vi "Main.vi"() -> ()   [LabVIEW 2017]
uses:
  type defs/action buttons.ctl
  type defs/mode buttons.ctl
  <vilib>/vision/Pattern Matching.llb/IMAQ GM Match Report.ctl
  type defs/states.ctl
  type defs/data.ctl
  <vilib>/vision/Image Controls.llb/IMAQ Image.ctl
  <vilib>/myRIO/Instrument Drivers/Onboard IO/PWM/typedefs/PWM Reference.ctl
  <vilib>/myRIO/Common/Instrument Driver Framework/Utilities/typedefs/myRIO Generic Hardware Reference.ctl
  <vilib>/myRIO/Common/Instrument Driver Framework/Utilities/typedefs/Hardware Version Enum.ctl
  <vilib>/myRIO/Common/Instrument Driver Framework/Utilities/typedefs/myRIO v1.0 Reference.ctl
  <vilib>/myRIO/Common/Instrument Driver Framework/Utilities/typedefs/Generic FPGA Reference.ctl
  <vilib>/myRIO/Common/Instrument Driver Framework/myRIO v1.0/PWM/typedefs/PWM Channels Enum.ctl
  <vilib>/myRIO/Instrument Drivers/Onboard IO/PWM/typedefs/PWM Configuration.ctl
  <vilib>/userdefined/High Color/nirio_resource_hc.ctl
  <vilib>/myRIO/Instrument Drivers/Onboard IO/DIO/typedefs/DIO Reference.ctl
  <vilib>/myRIO/Common/Instrument Driver Framework/myRIO v1.0/DIO/typedefs/DIO Channels List.ctl
  <vilib>/myRIO/Common/Instrument Driver Framework/myRIO v1.0/DIO/typedefs/DIO Channels Enum.ctl
  type defs/task.ctl
  <vilib>/myRIO/Common/Instrument Driver Framework/Utilities/vis/Is FPGA Ref Available.vi
  <vilib>/myRIO/Common/Instrument Driver Framework/myRIO v1.0/PWM/vis/myRIO v1.1 Open PWM.vi
  <vilib>/myRIO/Instrument Drivers/Onboard IO/PWM/vis/Set Duty Cycle and Frequency.vi
  <vilib>/myRIO/Common/Instrument Driver Framework/myRIO v1.0/DIO/vis/myRIO v1.1 Open DIO.vi
  <vilib>/myRIO/Instrument Drivers/Onboard IO/DIO/vis/Write.vi
  <vilib>/myRIO/Instrument Drivers/Onboard IO/DIO/vis/Read.vi
  <vilib>/myRIO/Common/Instrument Driver Framework/Utilities/vis/Validate Channels.vi
  <vilib>/myRIO/Common/Instrument Driver Framework/myRIO v1.0/PWM/vis/myRIO v1.0 Reserve PWM.vi
  <vilib>/myRIO/Common/Instrument Driver Framework/myRIO v1.0/DIO/vis/myRIO v1.0 Reserve DIO.vi
  <vilib>/myRIO/Common/Instrument Driver Framework/myRIO v1.0/UART/vis/myRIO v1.0 Close UART.vi
  <vilib>/myRIO/Common/Instrument Driver Framework/myRIO v1.0/PWM/vis/myRIO v1.0 Build MUX Configuration PWM.vi
  <vilib>/myRIO/Common/Instrument Driver Framework/myRIO v1.0/Resource Manager/vis/myRIO v1.0 Reserve Channel List.vi
  <vilib>/myRIO/Common/Instrument Driver Framework/myRIO v1.0/DIO/vis/myRIO v1.0 Build MUX Configuration DIO.vi
  <vilib>/myRIO/Common/Instrument Driver Framework/myRIO v1.0/Resource Manager/vis/myRIO v1.0 Create Configuration List.vi
  <vilib>/myRIO/Common/Instrument Driver Framework/myRIO v1.0/Resource Manager/vis/myRIO v1.0 Reserve Channel.vi
  <vilib>/myRIO/Common/Instrument Driver Framework/myRIO v1.0/Resource Manager/vis/myRIO v1.0 Unreserve Channel.vi
  <vilib>/myRIO/Common/Instrument Driver Framework/myRIO v1.0/Resource Manager/vis/myRIO v1.0 Build Mutex Name.vi
  <vilib>/Utility/VariantDataType/GetNumericInfo.vi
  <vilib>/Utility/error.llb/Error Cluster From Error Code.vi
  <vilib>/myRIO/Common/Instrument Driver Framework/myRIO v1.0/myRIO v1.1 Open.vi
  <vilib>/myRIO/Common/Instrument Driver Framework/Utilities/vis/IO Manager.vi
  <vilib>/myRIO/Common/Instrument Driver Framework/Utilities/vis/Configuration Manager.vi
  <vilib>/myRIO/Common/Instrument Driver Framework/myRIO v1.0/Resource Manager/vis/myRIO v1.0 Configure IO.vi
  <vilib>/myRIO/Common/Instrument Driver Framework/myRIO v1.0/myRIO v1.0 Close.vi
  <vilib>/myRIO/Common/Instrument Driver Framework/myRIO v1.0/PWM/vis/myRIO v1.0 Write PWM.vi
  <vilib>/myRIO/Common/Instrument Driver Framework/myRIO v1.0/DIO/vis/myRIO v1.0 Write DIO.vi
  <vilib>/myRIO/Common/Instrument Driver Framework/myRIO v1.0/DIO/vis/myRIO v1.0 Read DIO.vi
  <vilib>/myRIO/Common/Instrument Driver Framework/Utilities/vis/FPGA Ref Manager.vi
  <vilib>/myRIO/Common/Instrument Driver Framework/myRIO v1.0/myRIO v1.0 Reset FPGA.vi
  <vilib>/myRIO/Common/Instrument Driver Framework/myRIO v1.0/IRQ/vis/myRIO v1.0 IRQ Info FGV.vi
  <vilib>/myRIO/Common/Instrument Driver Framework/myRIO v1.0/IRQ/vis/myRIO v1.0 Timer IRQ Info FGV.vi
  <vilib>/myRIO/Common/Instrument Driver Framework/myRIO v1.0/IRQ/vis/myRIO v1.0 ISR Agent.vi
  <vilib>/myRIO/Express VI/Onboard IO/PWM/PWM Express VI.xnode
  <vilib>/myRIO/Instrument Drivers/Onboard IO/PWM/vis/myRIO PWM Open.xnode
  <vilib>/myRIO/Express VI/Onboard IO/DO/DO Express VI.xnode
  <vilib>/myRIO/Instrument Drivers/Onboard IO/DIO/vis/myRIO DIO Open.xnode
  <vilib>/myRIO/Express VI/Onboard Devices/LED/LED Express VI.xnode
  <vilib>/myRIO/Express VI/Onboard Devices/Button/Button Express VI.xnode
  <vilib>/vision/NI_Vision_Development_Module.lvlib
  <vilib>/myRIO/Instrument Drivers/Onboard IO/DIO/DIO.lvlib
  <vilib>/myRIO/Instrument Drivers/Onboard IO/PWM/PWM.lvlib
  <vilib>/myRIO/Instrument Drivers/Utilities/Utilities.lvlib
panel:
  in  "ROI Descriptor COLOR":T1={"Global Rectangle"=[86, 71, 180, 164], "Contours"=[{"ID"=enum."External", "Type"=3, "Coordinates"=[86, 71, 180, 164]}]} {"Contours"."Type" items=["No Selection", "Point", "Line", "Rectangle", "Oval", "Polygon", "Freehand Region", "Annulus", "Unused2", "Unused3", "Broken Line", "Freehand Line", "Rotated Rectangle"]}
  out "y0 (circle)":i32
  out "x0 (circle)":i32
  out "x1 (circle)":i32
  out "y1 (circle)":i32
  in  "divider (circle)":dbl=1.0
  out "error out 2":errorcluster
  out "___Test___":i32[](array[numeric])
  in  "Ball index":i32=1
  out "CircleRadius":dbl
  in  "Look at ball":bool
  in  "x = y?":bool
  in  "y":sgl=1.0
  out "Scale":sgl
  out "error out":errorcluster
  in  "Tab Control":enum32{"Motors", "Shape/Color", "Pattern"}(tab)
  in  "Left+":bool
  in  "Left-":bool
  in  "Right+":bool
  in  "Right-":bool
  in  "M+":bool
  in  "M-":bool
  in  "G+":bool
  in  "G-":bool
  in  "M_PWM":dbl=0.5
  in  "L_PWM":dbl=0.5
  in  "R_PWM":dbl=0.5
  in  "M+ (onGrab)":bool
  out "Circles Calibrated (Shape Detection 1)":T2(array[cluster]) {"Position"."Y" format="%.2f"; "Position"."X" format="%.2f"}
  out "Number of Matches (Shape Detection 1)":i32
  out "Color":i32
  in  "Circle Descriptor (Shape Detection 1)":cluster{"Min Radius":dbl, "Max Radius":dbl}={"Min Radius"=16.0, "Max Radius"=500.0}
  in  "Align X - t, Y - f":bool
  in  "grab time (ms)":u32
  out "Class (Particle Classification 1)":string
  out "y0":i32
  out "x0":i32
  out "x1":i32
  out "y1":i32
  out "Number of Matches (Geometric Matching 1)":i32
  out "Calibrated Matches (Geometric Matching 1)":T3[](array[typedef]) {"Correlation Score" format="%.2f"; "Target Template Curve Score" format="%.2f"; "Template Target Curve Score" format="%.2f"; "Bounding Box"."y" format="%.2f"; "Bounding Box"."x" format="%.2f"; "Position"."y" format="%.2f"; "Position"."x" format="%.2f"; "Score" format="%.2f"; "Scale" format="%.2f"; "Angle" format="%.2f"; "Occlusion %" format="%.2f"}
  out "curY":dbl
  out "curX":dbl
  out "Y is in range":bool
  out "X is in range":bool
  in  "defY":dbl=170.0
  in  "Range":dbl=40.0
  in  "defX":dbl=150.0
  in  "mode buttons":T4
  out "image display":T5(plugin-control)
  in  "action buttons":T6
  in  "Stop":bool
  # "Machine\nVision\nApp"
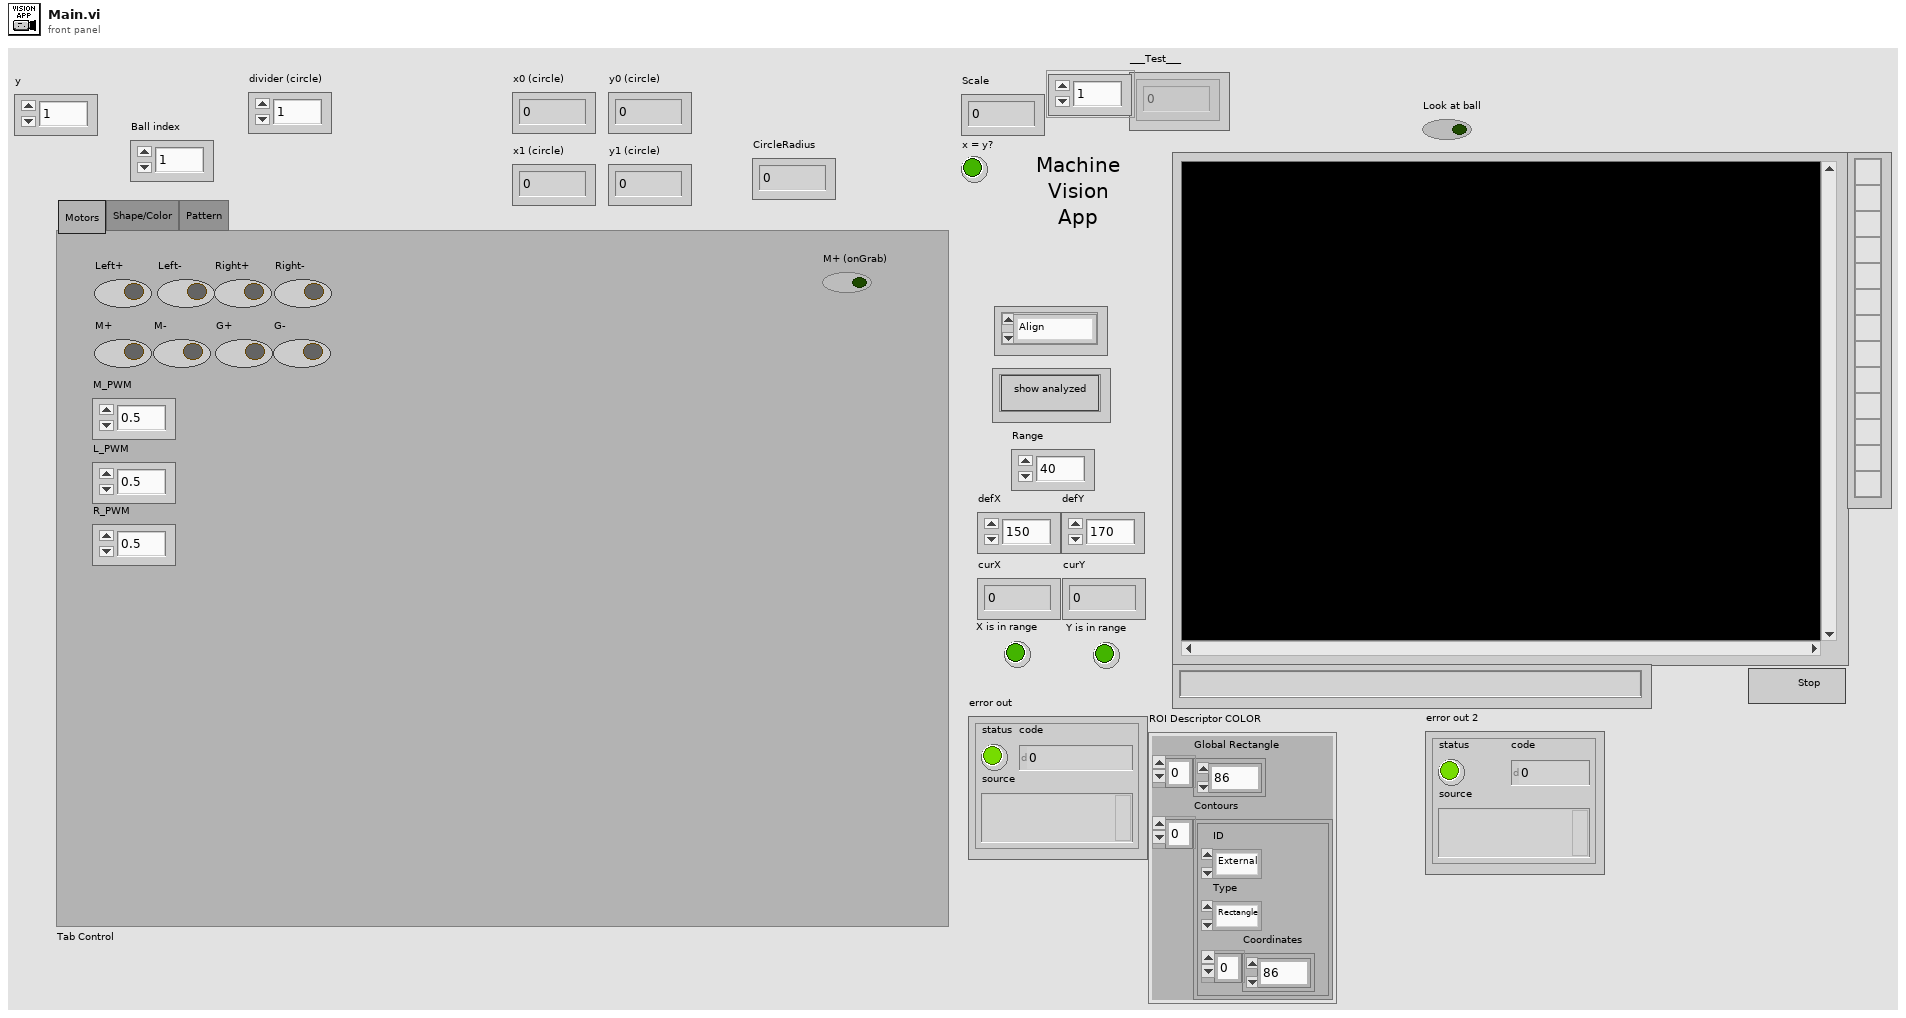
[diagram p1: front panel]
types:
  T1 = cluster{"Global Rectangle":i32[], "Contours":cluster{"ID":enum32{"External", "Internal"}, "Type":u32, "Coordinates":i32[]}[]}
  T2 = cluster{"Position":cluster{"X":sgl, "Y":sgl}, "Radius":dbl, "Score":dbl}[]
  T3 = typedef "IMAQ GM Match Report.ctl" = cluster{"Position":cluster{"x":sgl, "y":sgl}, "Angle":sgl, "Scale":sgl, "Score":sgl, "Bounding Box":cluster{"x":sgl, "y":sgl}[], "Contrast Reversed":bool, "Occlusion %":sgl, "Template Target Curve Score":sgl, "Target Template Curve Score":sgl, "Correlation Score":sgl}
  T4 = typedef "mode buttons.ctl" = cluster{"show analyzed":bool}
  T5 = typedef "IMAQ Image.ctl" = refnum<image>
  T6 = typedef "action buttons.ctl" = cluster{"Shape - t, Color - f":enum16{"Align", "Pattern", "Ball", "Other", "Clear", "Joystick control"}}
  T7 = typedef "data.ctl" = cluster{"Shape - t, Color - f":bool, "qsm":cluster{"Webcam image ref":T5, "Analyzed image ref":T5, "Stop webcam":bool}, " image ref":T5, "number img":i32, "ROI Descriptor (Image Mask 1)":cluster{"Global Rectangle":i32[], "Contours":cluster{"ID":enum32{"External", "Internal"}, "Type":u32, "Coordinates":i32[]}[]}, "Pattern class":i32, "Color class":i32, "ROI Descriptor COLOR Mask":cluster{"Global Rectangle":i32[], "Contours":cluster{"ID":enum32{"External", "Internal"}, "Type":u32, "Coordinates":i32[]}[]}, "___Test___":i32[]}
  T8 = typedef "states.ctl" = enum16{"(qsm) schedule", "(qsm) initialize", "(qsm) release", "(qsm) clean up", "(qsm) shutdown", "(myRIO) initialize", "(myRIO) clean up", "(myRIO) update ports", "(image) get", "(image) analyze", "(image) show", "(ball) Shape detection", "(ball) Calc ball indx", "(ball) Calculate ROI", "X align", "Wait", "Grab", "(pattern) Find Square", "(pattern) Calculate ROI", "(pattern) Analyze pattern", "(joystick) Joystick control", "Wait for button"}
  T9 = typedef "DIO.lvlib/DIO Reference.ctl" = cluster{"myRIO Reference":T10, "DIO Channels List":T14}
  T10 = typedef "myRIO Generic Hardware Reference.ctl" = cluster{"myRIO Model":T11, "myRIO Hardware Reference":T12}
  T11 = typedef "Hardware Version Enum.ctl" = enum16{"Unknown", "myRIO-1900", "myRIO-1950", "roboRIO", "NI ELVIS RIO CM"}
  T12 = typedef "myRIO v1.0 Reference.ctl" = cluster{"Generic FPGA Reference":T13, "Allow multiple opens":bool}
  T13 = typedef "Generic FPGA Reference.ctl" = refnum<k20>
  T14 = typedef "DIO Channels List.ctl" = T15[]
  T15 = typedef "DIO Channels Enum.ctl" = enum16{"Not Connected", "C/DIO0", "C/DIO1", "C/DIO2", "C/DIO3", "C/DIO4", "C/DIO5", "C/DIO6", "C/DIO7", "A/DIO0", "A/DIO1", "A/DIO2", "A/DIO3", "A/DIO4", "A/DIO5", "A/DIO6", "A/DIO7", "A/DIO8", "A/DIO9", "A/DIO10", "A/DIO11", "A/DIO12", "A/DIO13", "A/DIO14", "A/DIO15", "B/DIO0", "B/DIO1", "B/DIO2", "B/DIO3", "B/DIO4", "B/DIO5", "B/DIO6", "B/DIO7", "B/DIO8", "B/DIO9", "B/DIO10", "B/DIO11", "B/DIO12", "B/DIO13", "B/DIO14", "B/DIO15", "LED0", "LED1", "LED2", "LED3", "Button0", "DIO/DIO0", "DIO/DIO1", "DIO/DIO2", "DIO/DIO3", "DIO/DIO4", "DIO/DIO5", "DIO/DIO6", "DIO/DIO7", "DIO/DIO8", "DIO/DIO9", "SPI/CS0", "SPI/CS1", "SPI/CS2", "SPI/CS3", "LED RADIO (Green)", "LED RADIO (Red)", "LED COMM (Green)", "LED COMM (Red)", "LED MODE (Green)", "LED MODE (Red)"}
  T16 = typedef "nirio_resource_hc.ctl" = tag
  T17 = typedef "PWM.lvlib/PWM Reference.ctl" = cluster{"myRIO Reference":T10, "PWM Channels Enum":T18, "PWM Configuration":T19}
  T18 = typedef "PWM Channels Enum.ctl" = enum16{"Not Connected", "C/PWM0", "C/PWM1", "A/PWM0", "A/PWM1", "A/PWM2", "B/PWM0", "B/PWM1", "B/PWM2", "PWM/PWM0", "PWM/PWM1", "PWM/PWM2", "PWM/PWM3", "PWM/PWM4", "PWM/PWM5", "PWM/PWM6", "PWM/PWM7", "PWM/PWM8", "PWM/PWM9"}
  T19 = typedef "PWM.lvlib/PWM Configuration.ctl" = cluster{"Frequency":dbl, "Duty Cycle":dbl}
  T20 = enum16{"Align", "Pattern", "Ball", "Other", "Clear", "Joystick control"}
  T21 = typedef "task.ctl" = T8[]
  T22 = typedef "Image Type" = u32
  T23 = cluster{"Position":cluster{"X":sgl, "Y":sgl}, "Radius":dbl, "Score":dbl}
  T24 = cluster{"ID":enum32{"External", "Internal"}, "Type":u32, "Coordinates":i32[]}[]
  T25 = cluster{"ID":enum32{"External", "Internal"}, "Type":u32, "Coordinates":i32[]}
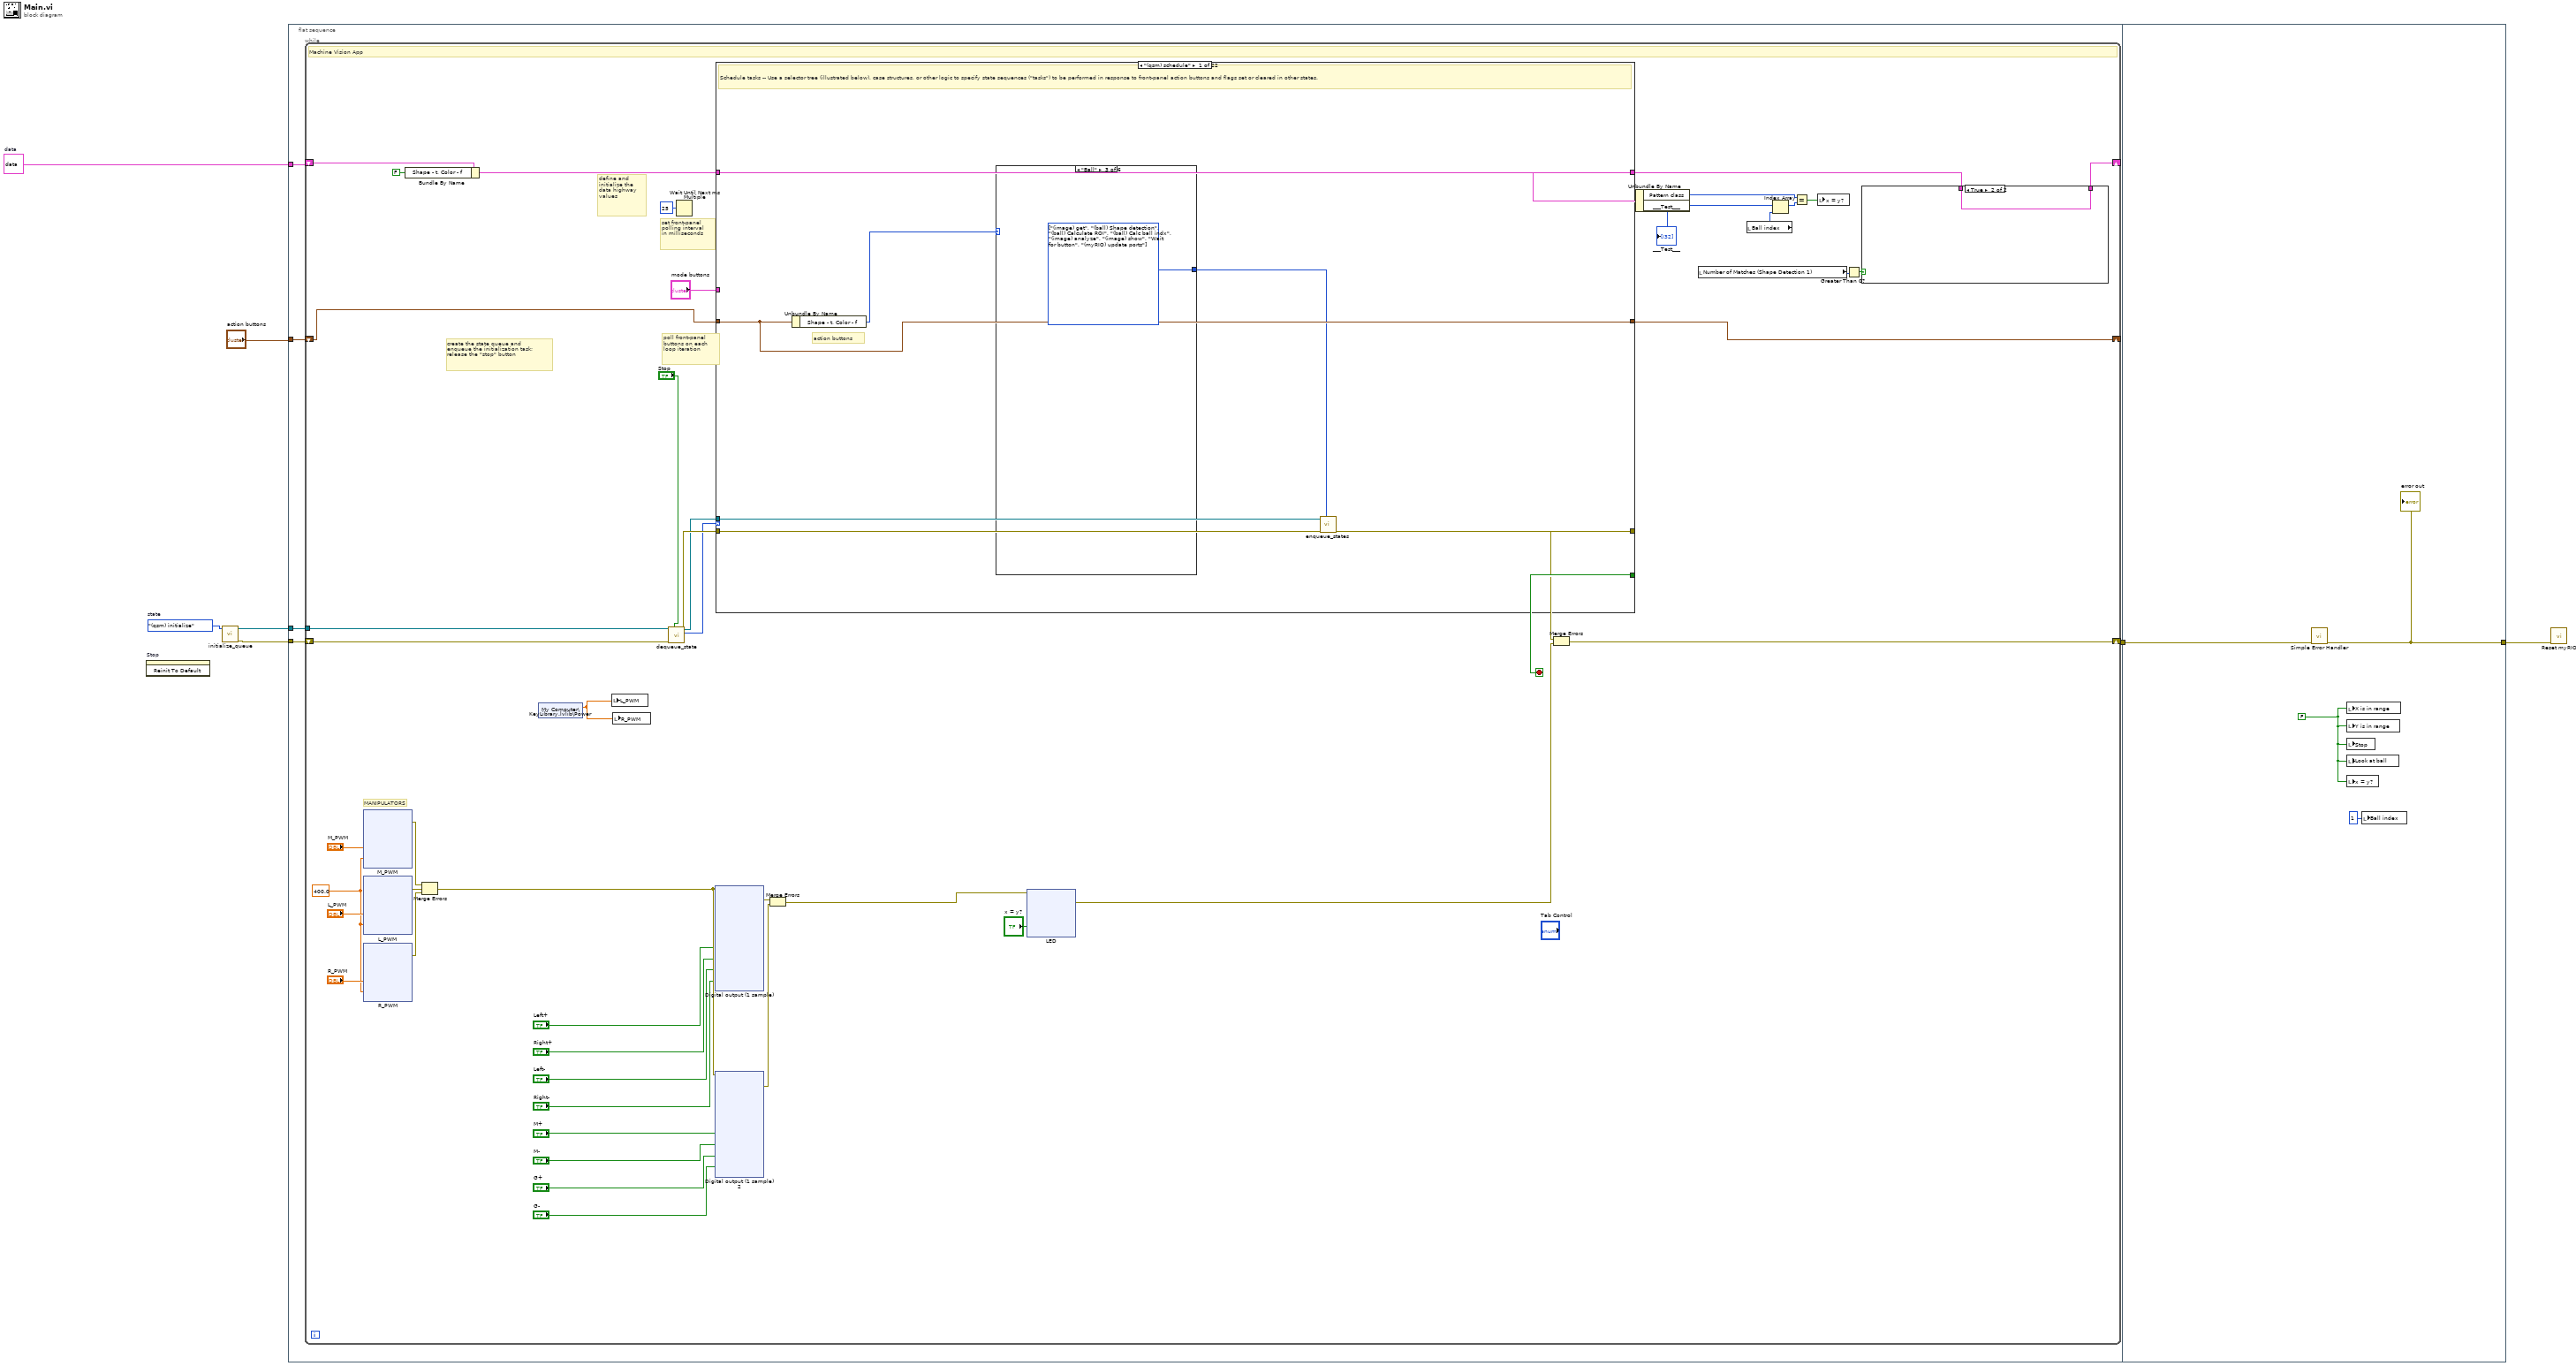
[diagram p0: block diagram]
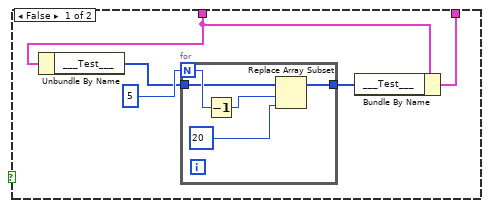
[diagram p2: hidden frame]
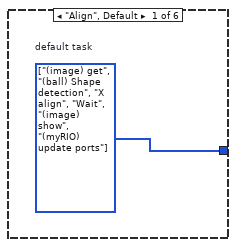
[diagram p3: hidden frame]
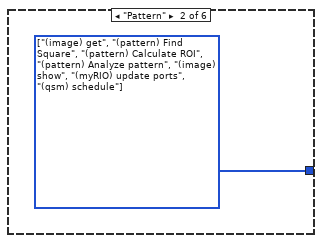
[diagram p4: hidden frame]
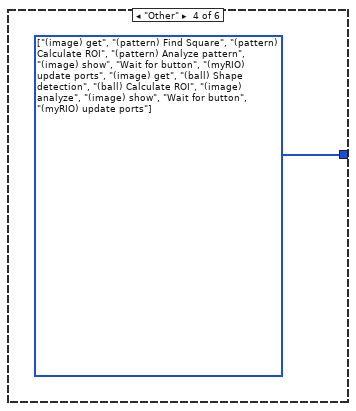
[diagram p5: hidden frame]
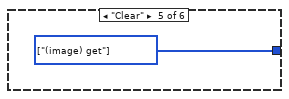
[diagram p6: hidden frame]
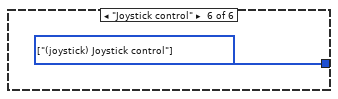
[diagram p7: hidden frame]
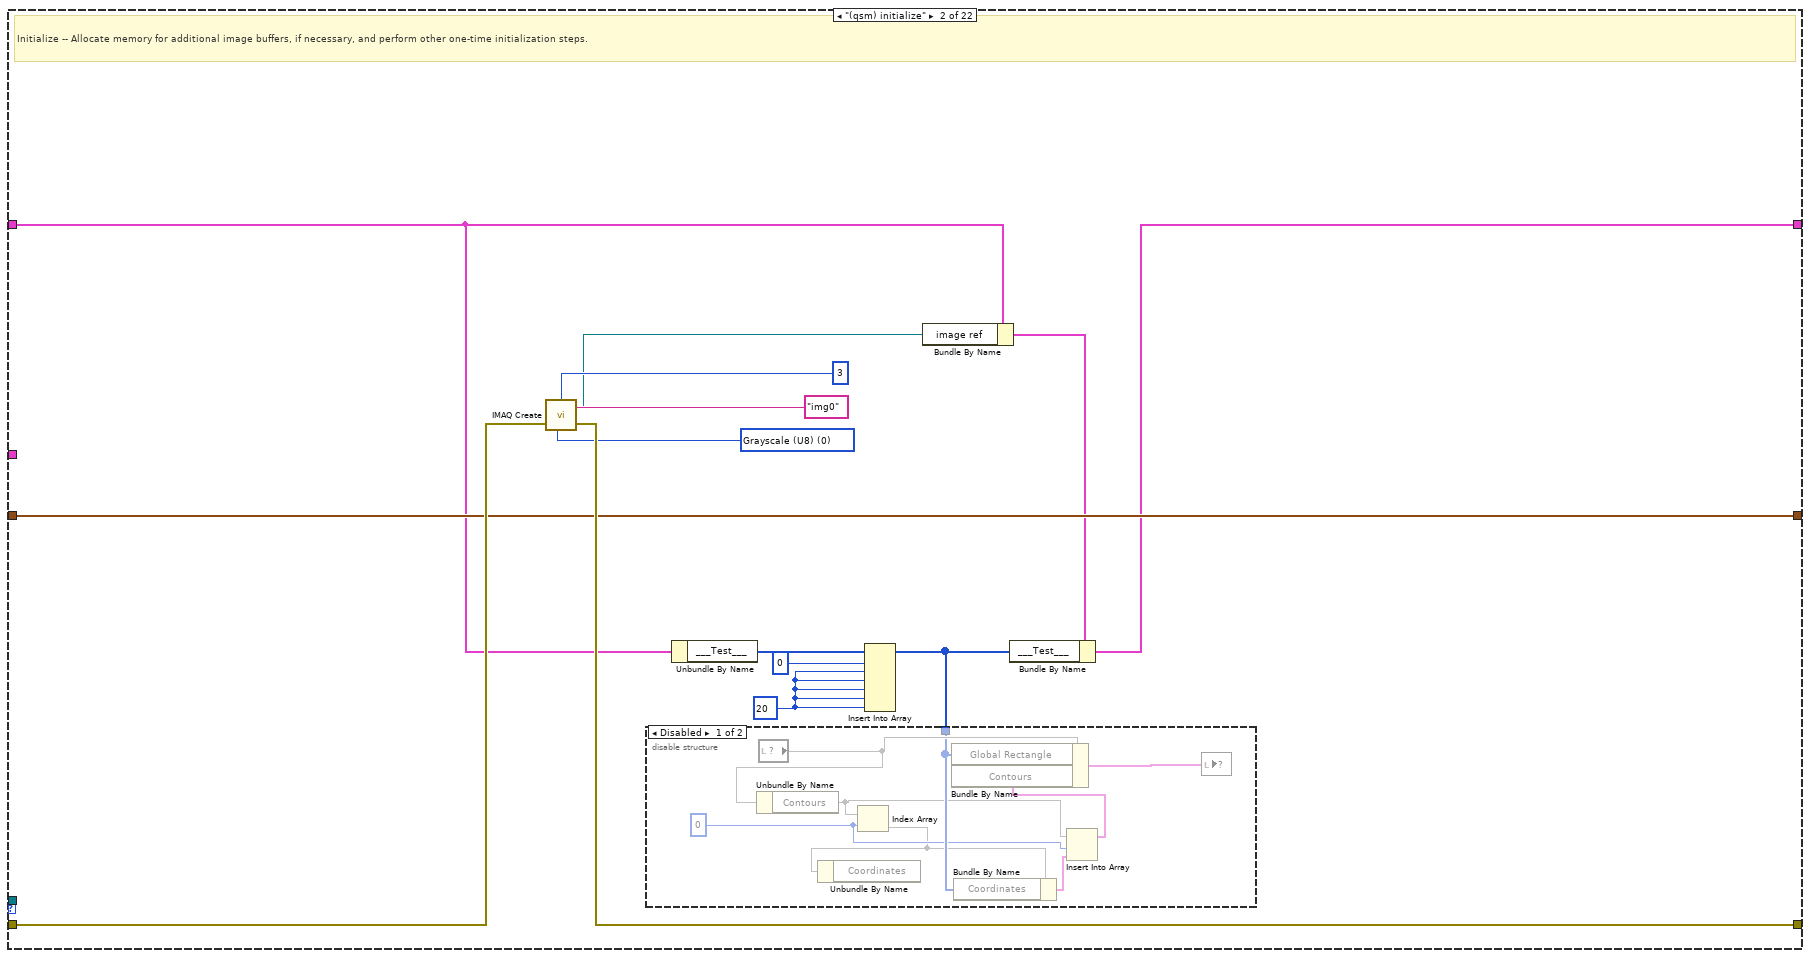
[diagram p8: hidden frame]
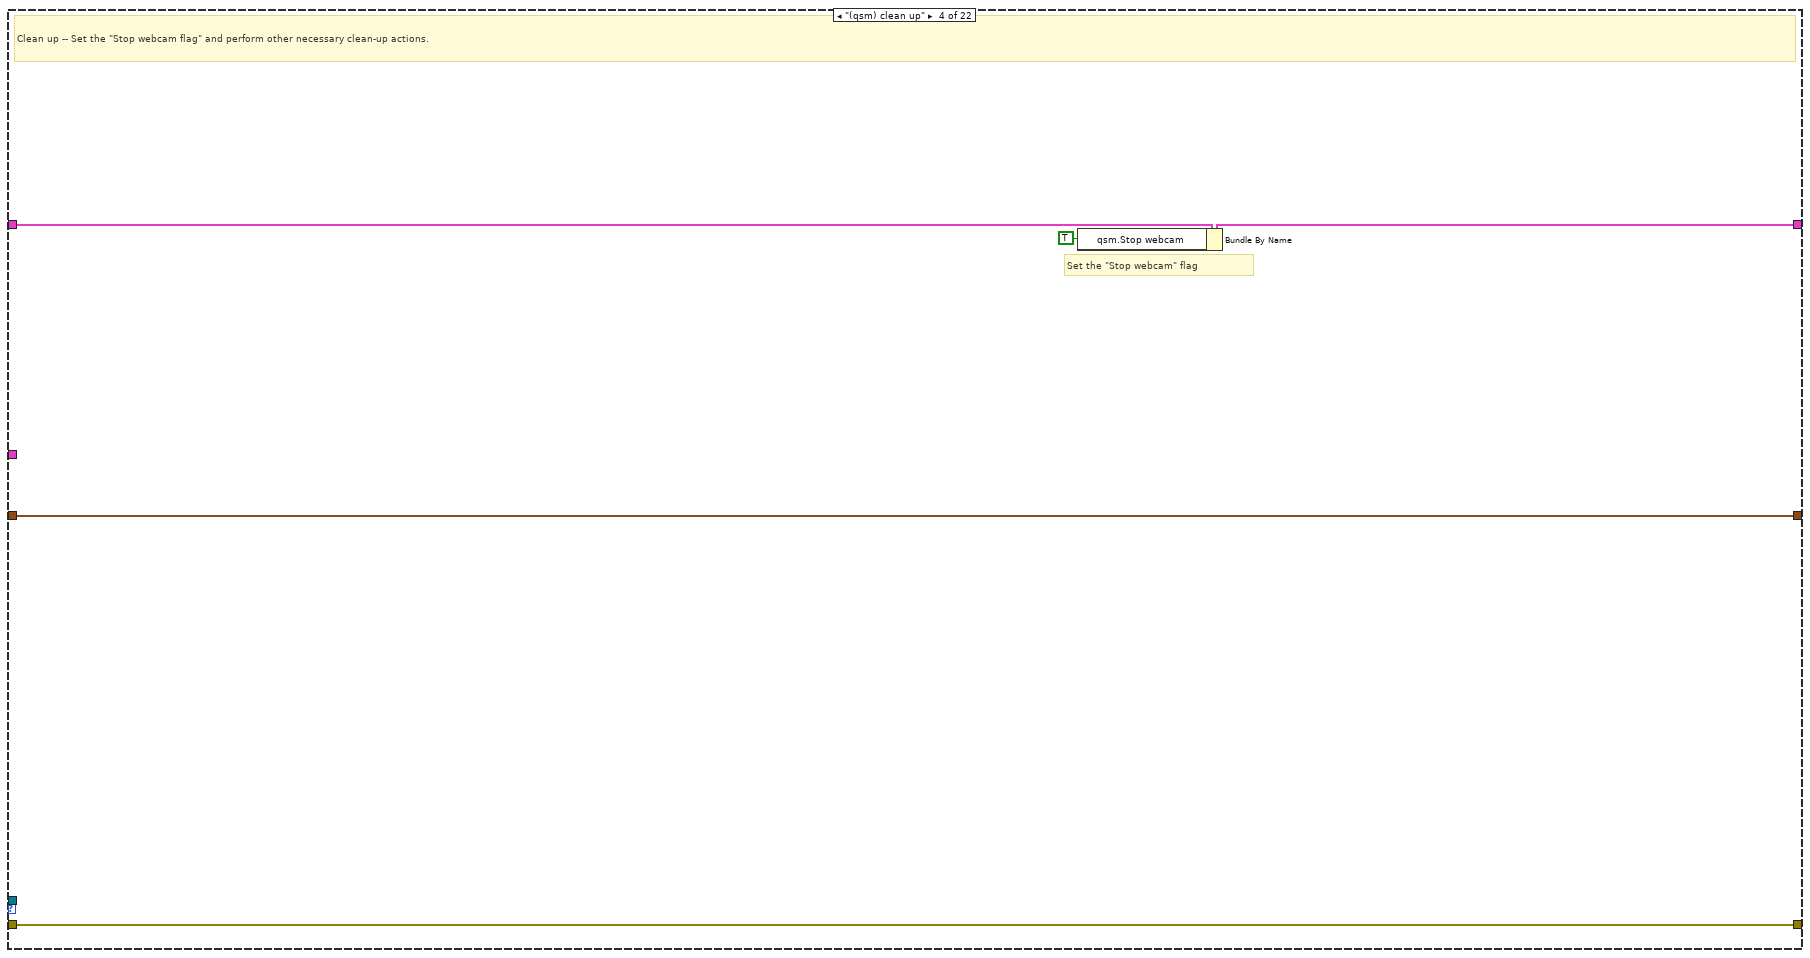
[diagram p11: hidden frame]
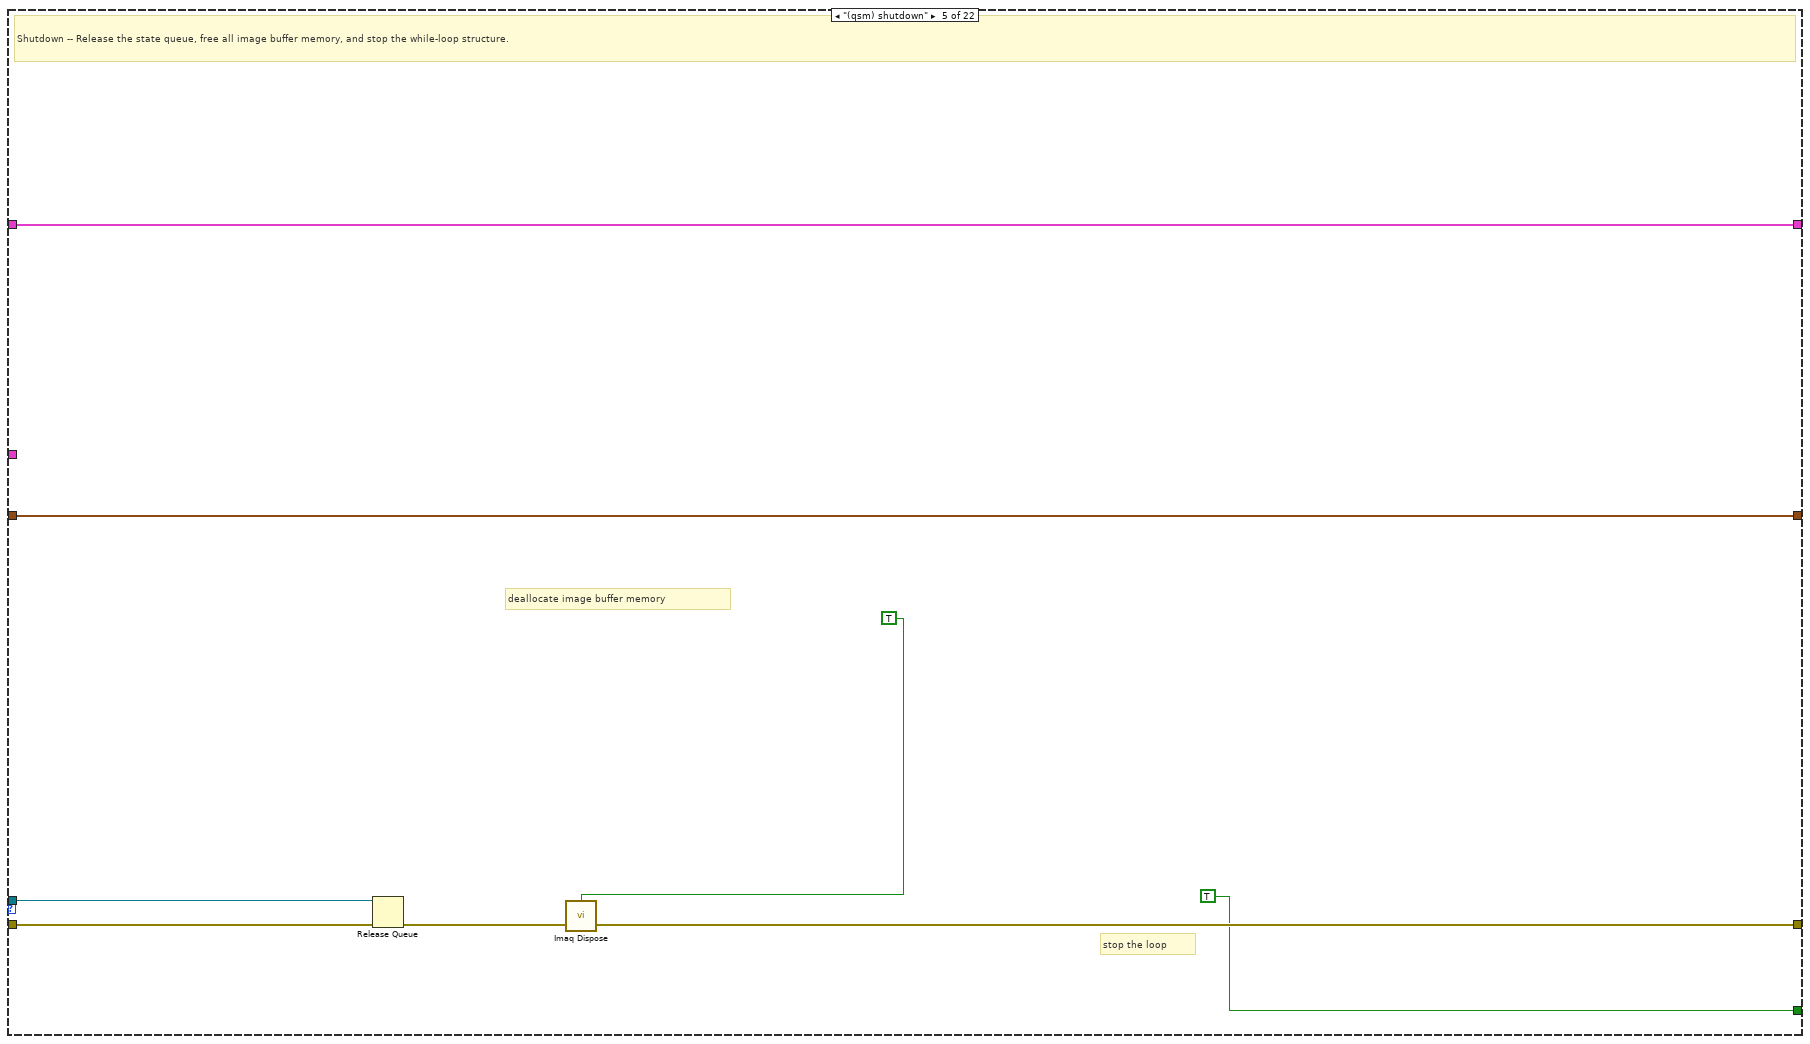
[diagram p12: hidden frame]
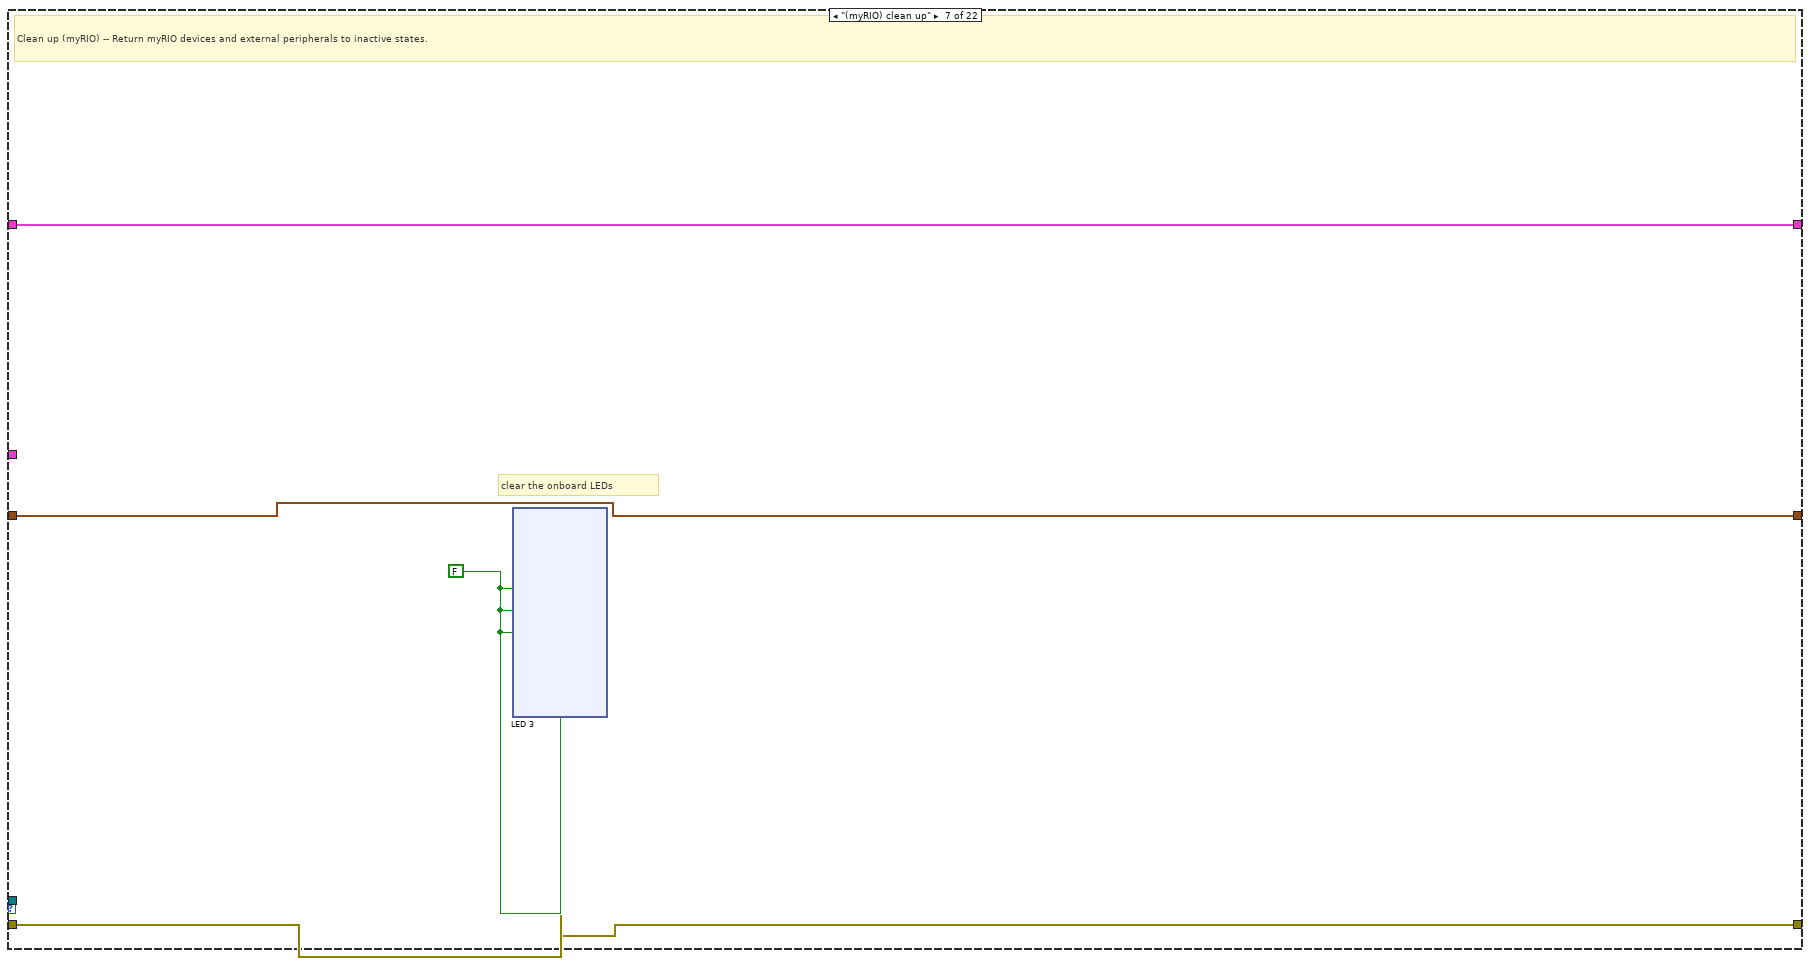
[diagram p14: hidden frame]
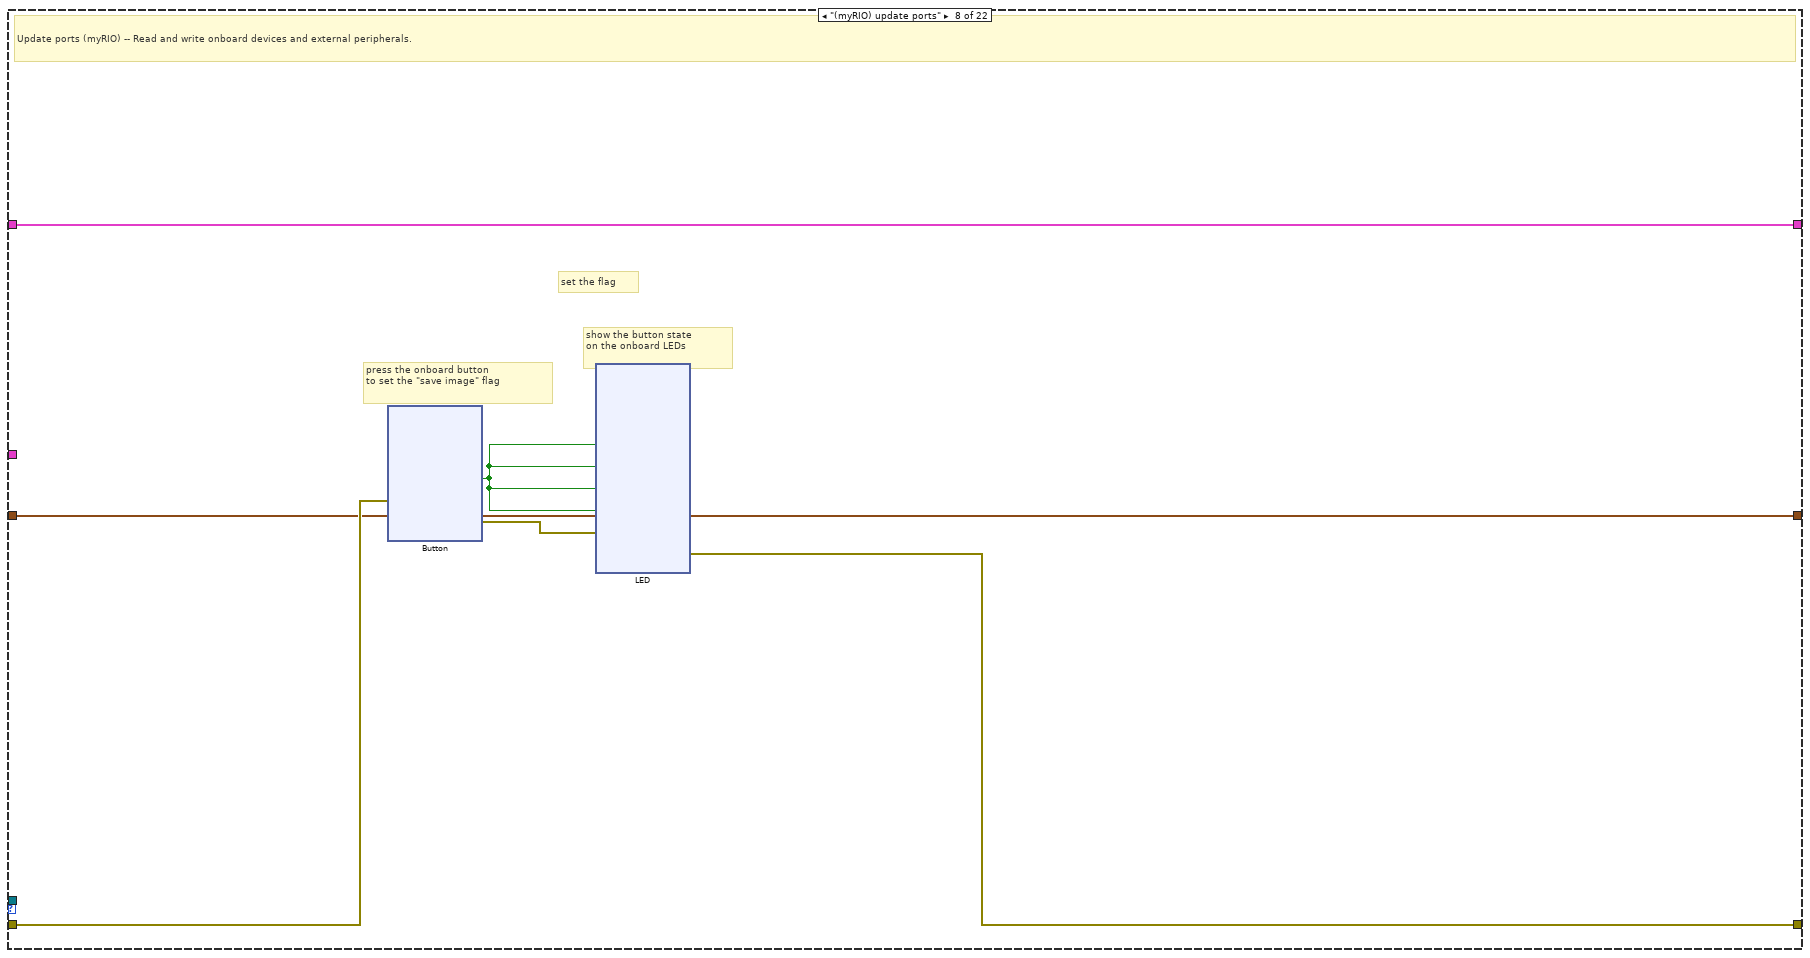
[diagram p15: hidden frame]
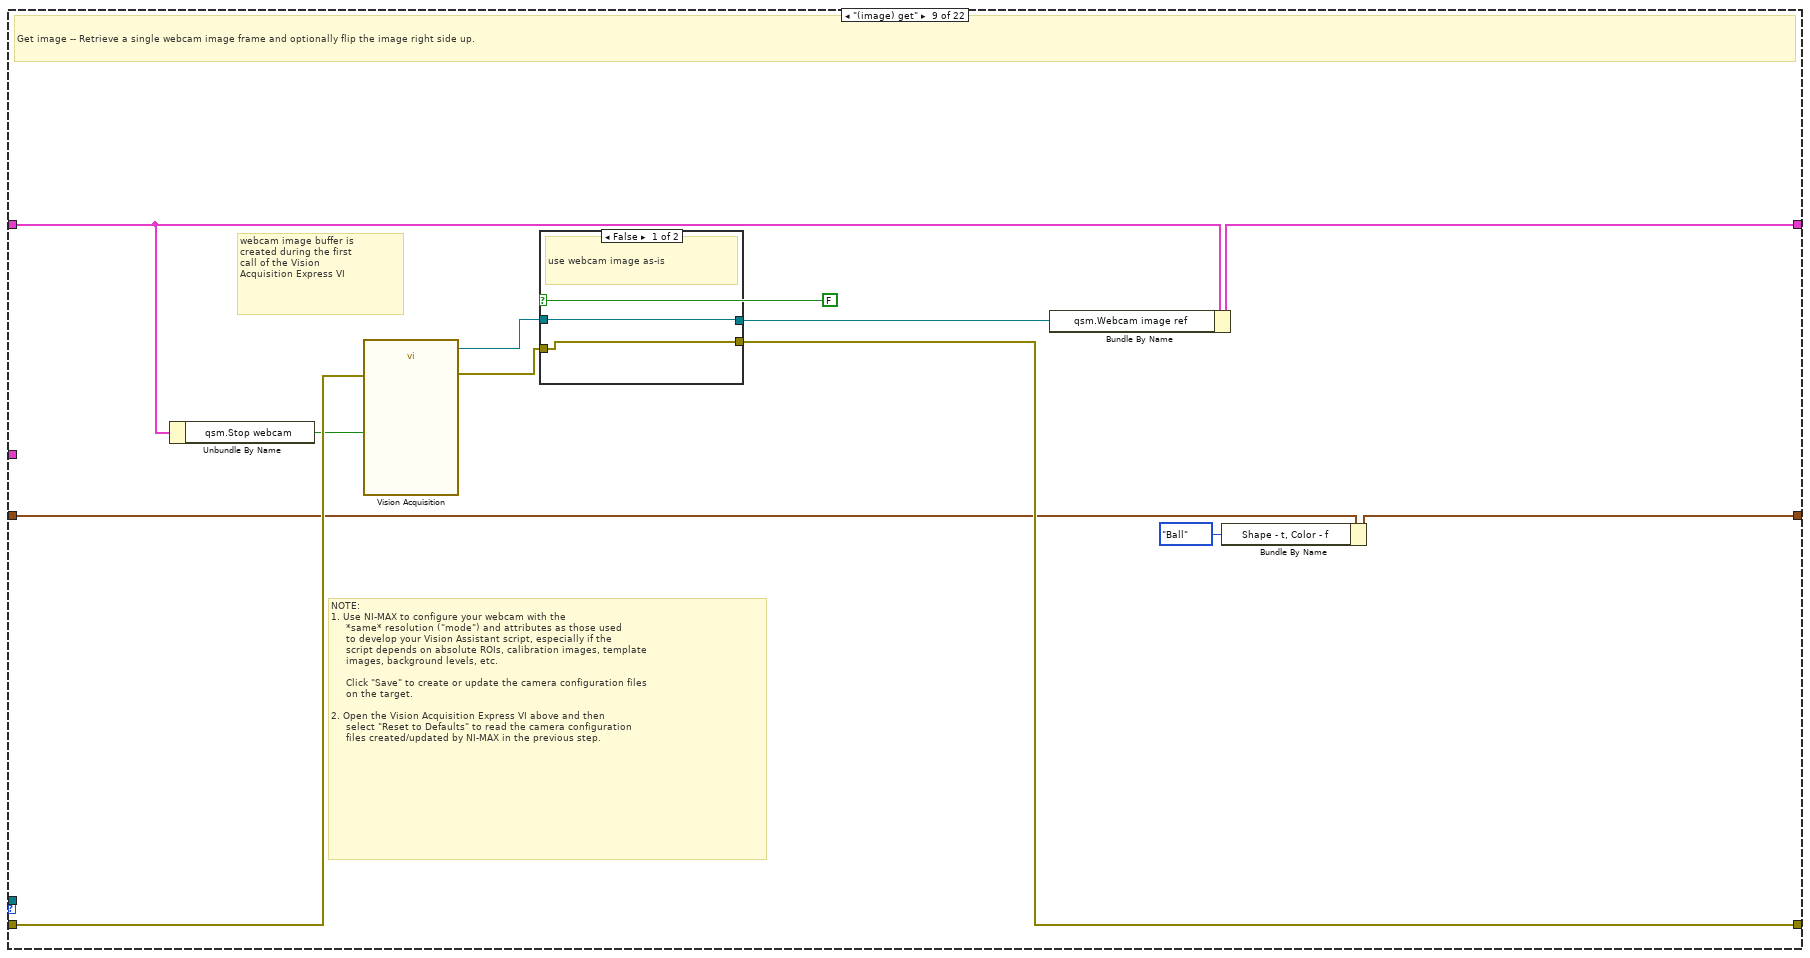
[diagram p16: hidden frame]
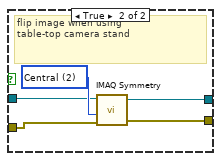
[diagram p17: hidden frame]
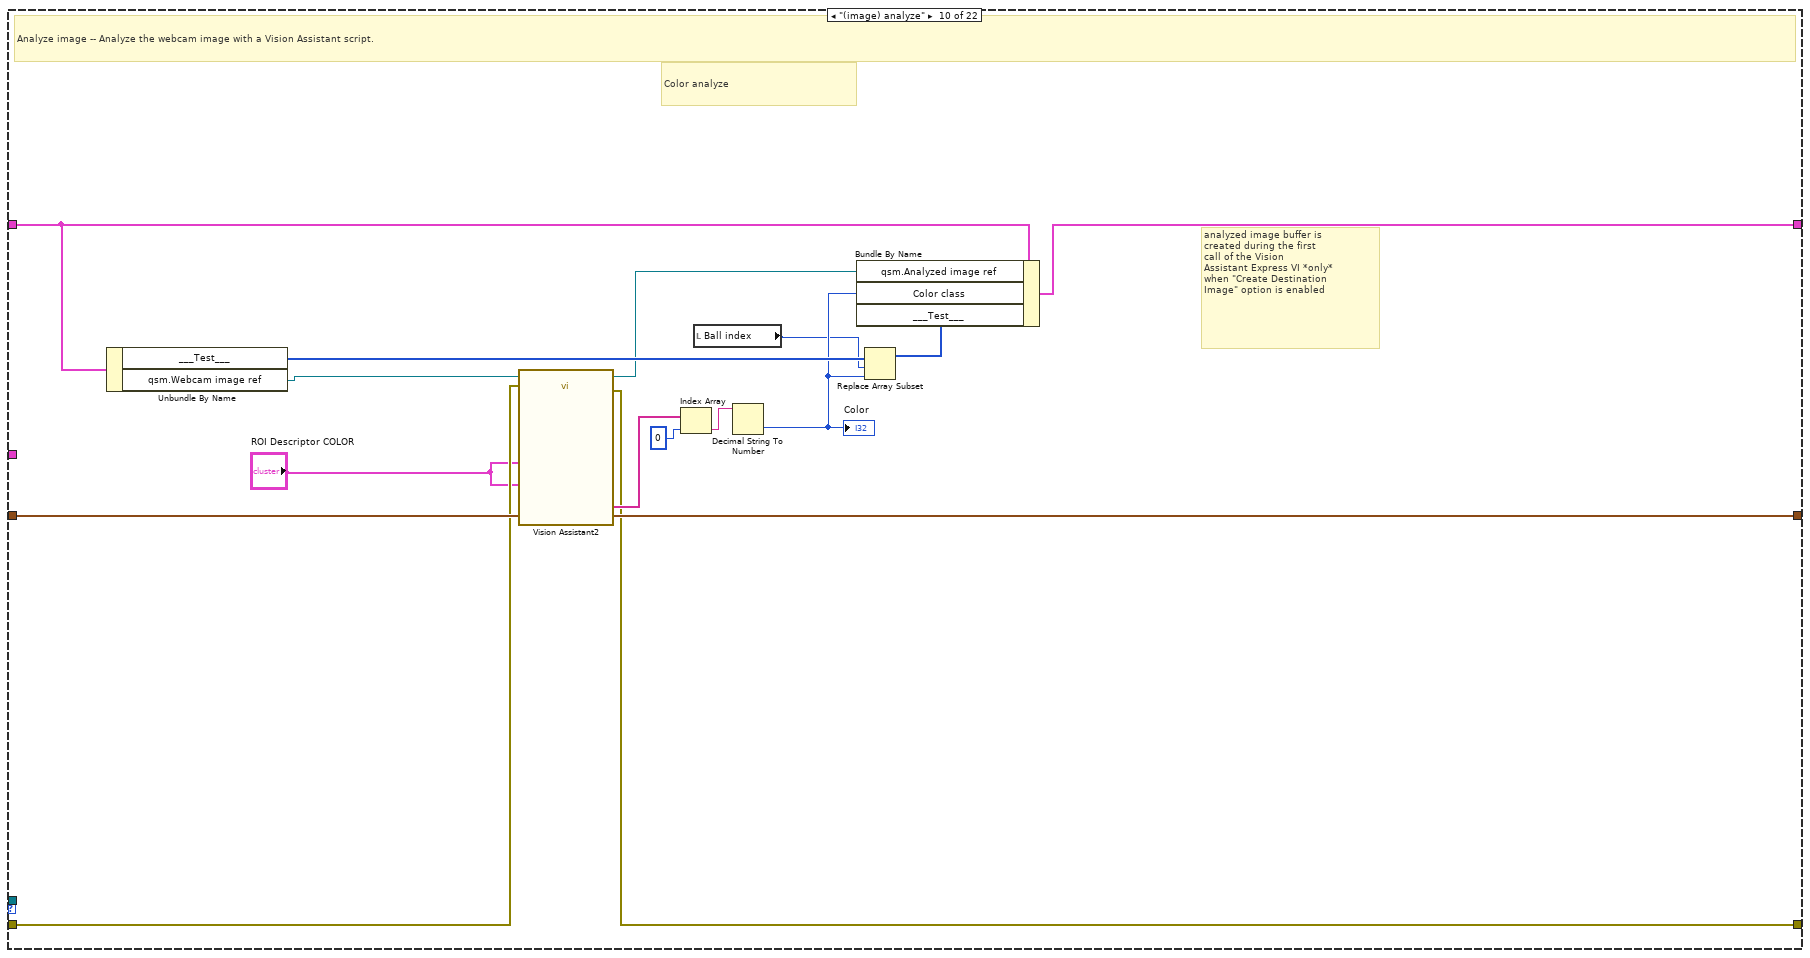
[diagram p18: hidden frame]
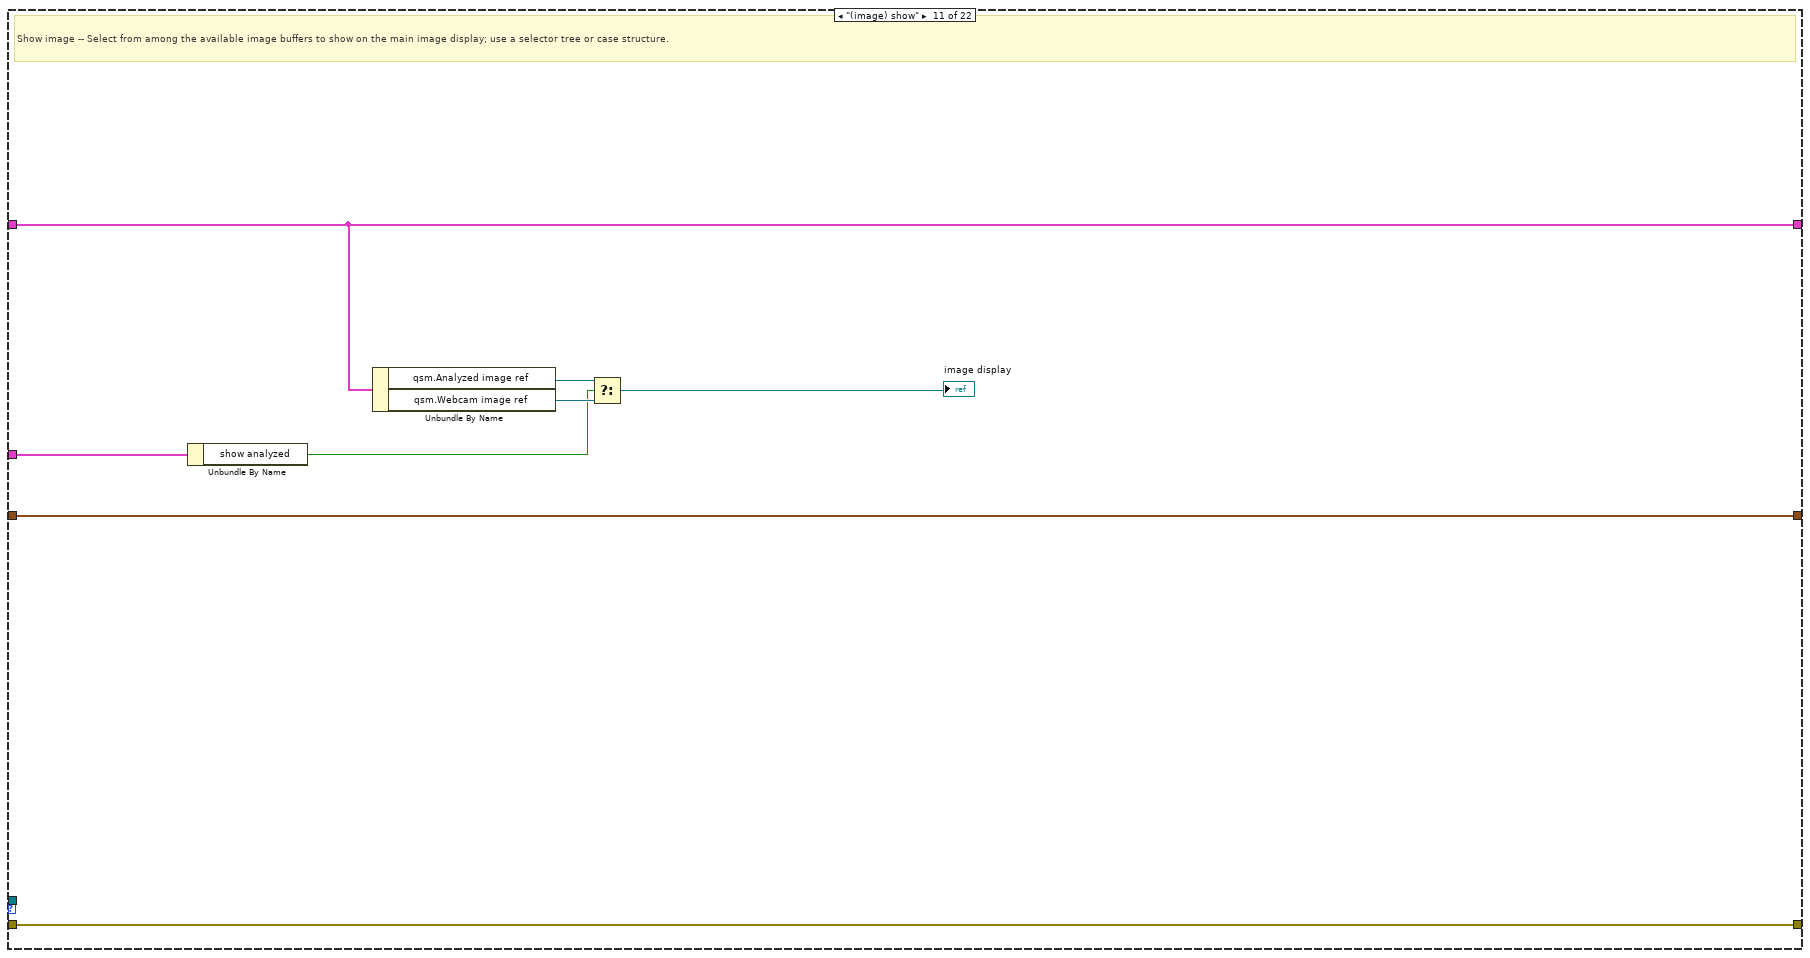
[diagram p19: hidden frame]
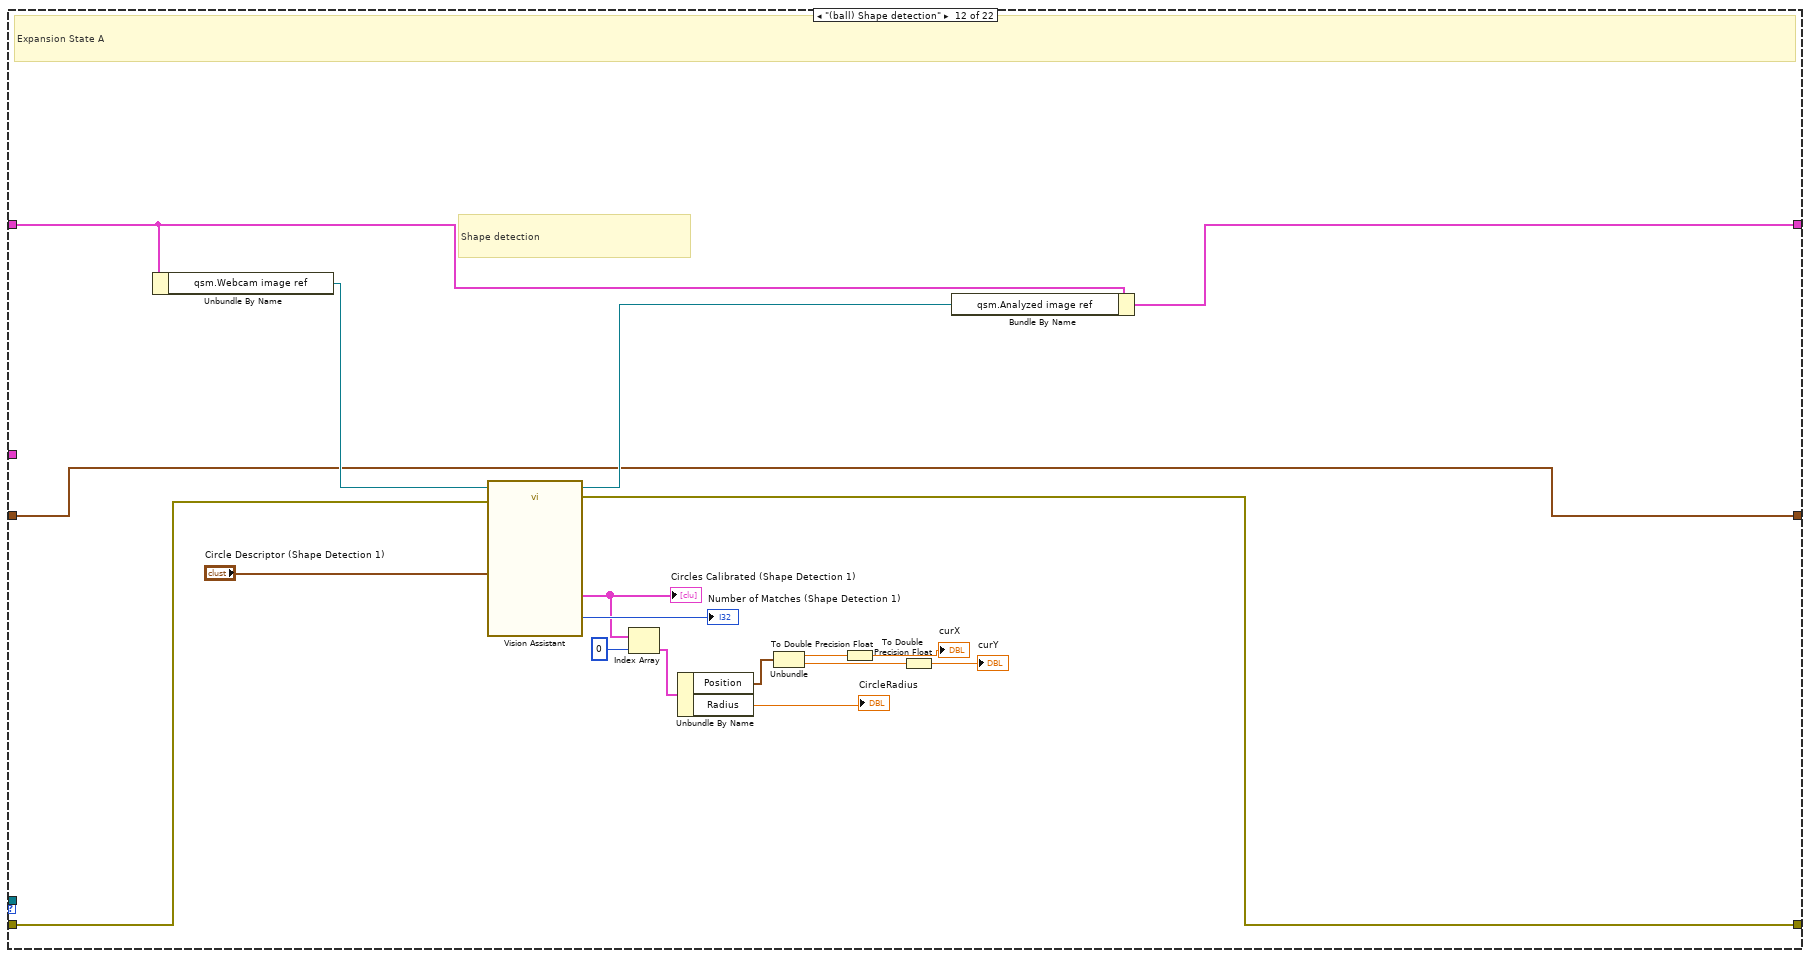
[diagram p20: hidden frame]
diagram:
  w1 = T7 {"Shape - t, Color - f"=FALSE, "qsm"={"Webcam image ref"=refnum, "Analyzed image ref"=refnum, "Stop webcam"=FALSE}, " image ref"=refnum, "number img"=0, "ROI Descriptor (Image Mask 1)"={"Global Rectangle"=[109, 72, 345, 284], "Contours"=[{"ID"=enum."External", "Type"=3, "Coordinates"=[109, 72, 345, 284]}]}, "Pattern class"=0, "Color class"=0, "ROI Descriptor COLOR Mask"={"Global Rectangle"=[51, 157, 345, 350], "Contours"=[{"ID"=enum."External", "Type"=5, "Coordinates"=[137, 230, 93, 226, 75, 199, 49, 200, 56, 145, 98, 111, 200, 119, 250, 126, 235, 166, 240, 212, 188, 243, 303, 244, 336, 247, 336, 271, 335, 292, 335, 318, 314, 323, 293, 334, 279, 345, 272, 349, 187, 349, 186, 335, 120, 334, 112, 314, 100, 297, 59, 291, 51, 288, 51, 287]}]}, "___Test___"=[]}  # data
  w2 = states."(qsm) initialize"  # state
  n1 = invoke on="Stop" class="Bool (strict)" method="Reinit To Default"() -> ()  [unwired: 3 in, 3 out]
  n2 = call "initialize_queue.vi"("state"=w2) -> ("error out"=w3:errorcluster, "queue out"=w4:refnum<queue>)  [unwired: 9 in]
  n3 = flat-sequence {
    tunnel: [w12] -> w6
    tunnel: "action buttons" -> [w11]
    tunnel: w3 -> [w9]
    tunnel: w4 -> [w10]
    tunnel: w1 -> [w8]
    tunnel: [w838] -> w7
    tunnel: w6 -> [w839]
    frame #0 {
      n4 = while {
        shift-right: [w53] -> w12
        shift-left: w9 -> [w58]
        shift-right: [w20] -> _
        shift-left: w8 -> [w34]
        shift-right: [w33] -> _
        shift-left: w11 -> [w32]
        tunnel: w10 -> [w31]
        stop <- w29 stop-if-true
        w36 = 400.0 ("Frequency [Hz]")
        # "define and \ninitialize the \ndata highway\nvalues"
        # "MANIPULATORS"
        # "create the state queue and\nenqueue the initialization task;\nrelease the \"stop\" button"
        # "set front-panel\npolling interval\nin milliseconds"
        # "poll front-panel\nbuttons on each\nloop iteration"
        # "Machine Vision App"
        n5 = xnode "M_PWM"("Duty Cycle"="M_PWM", "Frequency [Hz]"=w36) -> ("error out"=w52:errorcluster)  [unwired: 1 in]
        n6 = xnode "L_PWM"("Duty Cycle"="L_PWM", "Frequency [Hz]"=w36) -> ("error out"=w51:errorcluster)  [unwired: 1 in]
        n7 = xnode "R_PWM"("Duty Cycle"="R_PWM", "Frequency [Hz]"=w36) -> ("error out"=w50:errorcluster)  [unwired: 1 in]
        n8 = Bundle By Name(cluster=w34, "Shape - t, Color - f"=FALSE) -> (w28:T7)
        n9 = Merge Errors(w52, w51, w50) -> (w47:errorcluster)
        n10 = shared-variable "My Computer\\KeyLibrary.lvlib\\Power"() -> (w13:dbl)  [unwired: 1 in, 1 out]
        n11 = local write "L_PWM"(w13) -> ()
        n12 = local write "R_PWM"(w13) -> ()
        n13 = call "dequeue_state.vi"("stop"="Stop", "error in (no error)"=w58, "queue in"=w31) -> ("error out"=w59:errorcluster, "state"=w54:T8, "queue out"=w35:refnum<queue>)  [unwired: 6 in]
        n14 = Wait Until Next ms Multiple(millisecond multiple=u32 25) -> ()  [unwired: 1 out]
        n15 = xnode "Digital output (1 sample)"("Left+ (A/DIO5 (Pin 21))"="Left+", "Right+ (A/DIO7 (Pin 25))"="Right+", "Left- (A/DIO6 (Pin 23))"="Left-", "Right- (A/DIO13 (Pin 26))"="Right-", "error in (no error)"=w47) -> ("error out"=w49:errorcluster)
        n16 = xnode "Digital output (1 sample) 2"("M+ (B/DIO5 (Pin 21))"="M+", "M- (B/DIO6 (Pin 23))"="M-", "G+ (B/DIO7 (Pin 25))"="G+", "G- (B/DIO13 (Pin 26))"="G-", "error in (no error)"=w47) -> ("error out"=w48:errorcluster)
        n17 = case shown="\"(qsm) schedule\"" w54 {
          tunnel: w59 -> [w290 w313 w323 w326 w337 w339 w343 w388 w469 w484 w500 w522 w527 w543 w547 w583 w602 w685 w695 w751 w761 w832]
          tunnel: w35 -> [w291 _ _ _ w336 _ _ _ _ _ _ _ _ _ w546 w581 _ _ _ _ _ _]
          tunnel: [w292 w312 w323 w326 w332 w339 w342 w386 w472 w483 w500 w517 w527 w543 w547 w582 w601 w686 w695 w750 w760 w832] -> w17
          tunnel: w32 -> [w289 w307 w322 w325 w331 w338 w341 w384 w465 w493 w497 w513 w526 w541 w544 w585 w603 w690 w692 w746 w779 w833]
          tunnel: w28 -> [w293 w304 w324 w328 w335 w340 w345 w389 w470 w496 w501 w519 w528 w542 w548 w587 w604 w684 w693 w749 w780 w830]
          tunnel: [w293 w305 w324 w327 w335 w340 w345 w389 w474 w495 w501 w518 w528 w542 w548 w586 w604 w683 w694 w748 w780 w830] -> w21
          tunnel: "mode buttons" -> [_ _ _ _ _ _ _ _ _ _ w499 _ _ _ _ _ _ _ _ _ _ _]
          tunnel: [w289 w307 w322 w325 w331 w338 w341 w384 w464 w493 w497 w513 w526 w541 w544 w584 w603 w690 w692 w746 w779 w833] -> w33
          tunnel: [_ _ _ _ TRUE _ _ _ _ _ _ _ _ _ _ _ _ _ _ _ _ _] -> w29
          frame "(qsm) schedule" {
            # "action buttons"
            # "Schedule tasks -- Use a selector tree (illustrated below), case structures, or other logic to specify state sequences (\"tasks\") to be performed in response to front-panel action buttons and flags set or cleared in other states."
            n18 = Unbundle By Name(w289) -> ("Shape - t, Color - f"=w288:T20)
            n19 = case shown="\"Ball\"" w288 {
              tunnel: [w294 w295 w296 w297 w298 w299] -> w287
              frame "Align", Default {
                w294 = T21 [enum."(image) get", enum."(ball) Shape detection", enum."X align", enum."Wait", enum."(image) show", enum."(myRIO) update ports"] items=["(qsm) schedule", "(qsm) initialize", "(qsm) release", "(qsm) clean up", "(qsm) shutdown", "(myRIO) initialize", "(myRIO) clean up", "(myRIO) update ports", "(image) get", "(image) analyze", "(image) show", "(ball) Shape detection", "(ball) Calc ball indx", "(ball) Calculate ROI", "X align", "Wait", "Grab", "(pattern) Find Square", "(pattern) Calculate ROI", "(pattern) Analyze pattern", "(joystick) Joystick control", "Wait for button"]  # default task
              }
              frame "Pattern" {
                w295 = T21 [enum."(image) get", enum."(pattern) Find Square", enum."(pattern) Calculate ROI", enum."(pattern) Analyze pattern", enum."(image) show", enum."(myRIO) update ports", enum."(qsm) schedule"] items=["(qsm) schedule", "(qsm) initialize", "(qsm) release", "(qsm) clean up", "(qsm) shutdown", "(myRIO) initialize", "(myRIO) clean up", "(myRIO) update ports", "(image) get", "(image) analyze", "(image) show", "(ball) Shape detection", "(ball) Calc ball indx", "(ball) Calculate ROI", "X align", "Wait", "Grab", "(pattern) Find Square", "(pattern) Calculate ROI", "(pattern) Analyze pattern", "(joystick) Joystick control", "Wait for button"] ("task")
              }
              frame "Ball" {
                w296 = T21 [enum."(image) get", enum."(ball) Shape detection", enum."(ball) Calculate ROI", enum."(ball) Calc ball indx", enum."(image) analyze", enum."(image) show", enum."Wait for button", enum."(myRIO) update ports"] items=["(qsm) schedule", "(qsm) initialize", "(qsm) release", "(qsm) clean up", "(qsm) shutdown", "(myRIO) initialize", "(myRIO) clean up", "(myRIO) update ports", "(image) get", "(image) analyze", "(image) show", "(ball) Shape detection", "(ball) Calc ball indx", "(ball) Calculate ROI", "X align", "Wait", "Grab", "(pattern) Find Square", "(pattern) Calculate ROI", "(pattern) Analyze pattern", "(joystick) Joystick control", "Wait for button"] ("task")
              }
              frame "Other" {
                w297 = T21 [enum."(image) get", enum."(pattern) Find Square", enum."(pattern) Calculate ROI", enum."(pattern) Analyze pattern", enum."(image) show", enum."Wait for button", enum."(myRIO) update ports", enum."(image) get", enum."(ball) Shape detection", enum."(ball) Calculate ROI", enum."(image) analyze", enum."(image) show", enum."Wait for button", enum."(myRIO) update ports"] items=["(qsm) schedule", "(qsm) initialize", "(qsm) release", "(qsm) clean up", "(qsm) shutdown", "(myRIO) initialize", "(myRIO) clean up", "(myRIO) update ports", "(image) get", "(image) analyze", "(image) show", "(ball) Shape detection", "(ball) Calc ball indx", "(ball) Calculate ROI", "X align", "Wait", "Grab", "(pattern) Find Square", "(pattern) Calculate ROI", "(pattern) Analyze pattern", "(joystick) Joystick control", "Wait for button"] ("task")
              }
              frame "Clear" {
                w298 = T21 [enum."(image) get"] items=["(qsm) schedule", "(qsm) initialize", "(qsm) release", "(qsm) clean up", "(qsm) shutdown", "(myRIO) initialize", "(myRIO) clean up", "(myRIO) update ports", "(image) get", "(image) analyze", "(image) show", "(ball) Shape detection", "(ball) Calc ball indx", "(ball) Calculate ROI", "X align", "Wait", "Grab", "(pattern) Find Square", "(pattern) Calculate ROI", "(pattern) Analyze pattern", "(joystick) Joystick control", "Wait for button"]
              }
              frame "Joystick control" {
                w299 = T21 [enum."(joystick) Joystick control"] items=["(qsm) schedule", "(qsm) initialize", "(qsm) release", "(qsm) clean up", "(qsm) shutdown", "(myRIO) initialize", "(myRIO) clean up", "(myRIO) update ports", "(image) get", "(image) analyze", "(image) show", "(ball) Shape detection", "(ball) Calc ball indx", "(ball) Calculate ROI", "X align", "Wait", "Grab", "(pattern) Find Square", "(pattern) Calculate ROI", "(pattern) Analyze pattern", "(joystick) Joystick control", "Wait for button"]
              }
            }
            n20 = call "enqueue_states.vi"("task"=w287, "error in"=w290, "queue in"=w291) -> ("error out"=w292:errorcluster)  [unwired: 6 in, 1 out]
          }
          frame "(qsm) initialize" {
            w301 = 20
            w310 = T22 0 items=["Grayscale (U8)", "Grayscale (I16)", "Grayscale (SGL)", "Complex (CSG)", "RGB (U32)", "HSL (U32)", "RGB (U64)", "Grayscale (U16)"] ("Image Type")
            # "Initialize -- Allocate memory for additional image buffers, if necessary, and perform other one-time initialization steps."
            n21 = call "IMAQ Create"("Border Size"=3, "Image Name"="img0", "Image Type"=w310, "error in (no error)"=w313) -> ("New Image"=w308:T5, "error out"=w312:errorcluster)  [unwired: 1 in]
            n22 = Unbundle By Name(w304) -> ("___Test___"=w302:i32[])
            n23 = Insert Into Array(array=w302, index=0, new element #1=w301, new element #2=w301, new element #3=w301, new element #4=w301, new element #5=w301) -> (w300:i32[])
            n24 = disable-structure shown="Disabled" {
              disable-tunnel: w300 -> [w319 _]
              frame Disabled {
                w318 = 0 ("index")
                n25 = local read item#-1() -> (w320)
                n26 = Unbundle By Name(w320) -> ("Contours"=w317)
                n27 = Index Array(array=w317, index=w318) -> (element=w316)
                n28 = Unbundle By Name(w316) -> ()  [unwired: 1 out]
                n29 = Bundle By Name(cluster=w316, "Coordinates"=w319) -> (w315:cluster{})
                n30 = Insert Into Array(array=w317, index=w318, new element=w315) -> (w314:cluster{}[])
                n31 = Bundle By Name(cluster=w320, "Global Rectangle"=w319, "Contours"=w314) -> (w321:cluster{})
                n32 = local write item#-1(w321) -> ()
              }
              frame Enabled {
              }
            }
            n33 = Bundle By Name(cluster=w304, "image ref"=w308) -> (w306:T7)
            n34 = Bundle By Name(cluster=w306, "___Test___"=w300) -> (w305:T7)
          }
          frame "(qsm) release" {
            # "Release all front-panel action buttons."
          }
          frame "(qsm) clean up" {
            # "Set the \"Stop webcam\" flag"
            # "Clean up -- Set the \"Stop webcam flag\" and perform other necessary clean-up actions."
            n35 = Bundle By Name(cluster=w328, "qsm.Stop webcam"=TRUE) -> (w327:T7)
          }
          frame "(qsm) shutdown" {
            # "deallocate image buffer memory"
            # "stop the loop"
            # "Shutdown -- Release the state queue, free all image buffer memory, and stop the while-loop structure."
            n36 = Release Queue(queue=w336, error in (no error)=w337) -> (error out=w333:errorcluster)  [unwired: 1 in, 2 out]
            n37 = call "Imaq Dispose"("All Images? (No)"=TRUE, "error in (no error)"=w333) -> ("error out"=w332:errorcluster)  [unwired: 4 in]
          }
          frame "(myRIO) initialize" {
            # "Initialize (myRIO) -- Open channels, configure devices, send setup strings to peripherals, etc."
          }
          frame "(myRIO) clean up" {
            w344 = FALSE ("LED3")
            # "clear the onboard LEDs"
            # "Clean up (myRIO) -- Return myRIO devices and external peripherals to inactive states."
            n38 = xnode "LED 3"("LED0"=w344, "LED1"=w344, "LED2"=w344, "LED3"=w344, "error in (no error)"=w343) -> ("error out"=w342:errorcluster)
          }
          frame "(myRIO) update ports" {
            # "show the button state\non the onboard LEDs"
            # "set the flag"
            # "press the onboard button\nto set the \"save image\" flag"
            # "Update ports (myRIO) -- Read and write onboard devices and external peripherals."
            n39 = xnode "Button"("error in (no error)"=w388) -> ("Value"=w385:bool, "error out"=w387:errorcluster)
            n40 = xnode "LED"("LED0"=w385, "LED1"=w385, "LED2"=w385, "LED3"=w385, "error in (no error)"=w387) -> ("error out"=w386:errorcluster)
          }
          frame "(image) get" {
            # "NOTE:\n1. Use NI-MAX to configure your webcam with the\n     *same* resolution (\"mode\") and attributes as those used \n     to develop your Vision Assistant script, especially if the\n     script depends on absolute ROIs, calibration images, template\n     images, background levels, etc.\n \n     Click \"Save\" to create or update the camera configuration files\n     on the target.\n\n2. Open the Vision Acquisition Express VI above and then\n     select \"Reset to Defaults\" to read the camera configuration\n     files created/updated by NI-MAX in the previous step."
            # "webcam image buffer is\ncreated during the first\ncall of the Vision\nAcquisition Express VI"
            # "Get image -- Retrieve a single webcam image frame and optionally flip the image right side up."
            n41 = Unbundle By Name(w470) -> ("qsm.Stop webcam"=w468:bool)
            n42 = call "Vision Acquisition"("Stop (F)"=w468, "error in"=w469) -> ("Image Out"=w467:T5, "error out"=w466:errorcluster)  [unwired: 22 in, 2 out]
            n43 = case shown="False" FALSE {
              tunnel: w467 -> [w476 w480]
              tunnel: [w476 w479] -> w473
              tunnel: w466 -> [w475 w478]
              tunnel: [w475 w477] -> w472
              frame False {
                # "use webcam image as-is"
              }
              frame True {
                w481 = u32 2 items=["Horizontal", "Vertical", "Central", "1st Diagonal", "2nd Diagonal"] ("Type of Symmetry")
                # "flip image when using\ntable-top camera stand"
                n44 = call "IMAQ Symmetry"("error in (no error)"=w478, "Type of Symmetry"=w481, "Image Src"=w480) -> ("error out"=w477:errorcluster, "Image Dst Out"=w479:T5)  [unwired: 2 in]
              }
            }
            n45 = Bundle By Name(cluster=w470, "qsm.Webcam image ref"=w473) -> (w474:T7)
            n46 = Bundle By Name(cluster=w465, "Shape - t, Color - f"=T20."Ball") -> (w464:T6)
          }
          frame "(image) analyze" {
            # "Color analyze"
            # "analyzed image buffer is\ncreated during the first\ncall of the Vision\nAssistant Express VI *only*\nwhen \"Create Destination\nImage\" option is enabled"
            # "Analyze image -- Analyze the webcam image with a Vision Assistant script."
            n47 = Unbundle By Name "Unbundle By Name"(w496) -> ("___Test___"=w490:i32[], "qsm.Webcam image ref"=w487:T5)
            n48 = call "Vision Assistant2"("Image In"=w487, "error in"=w484, "ROI Descriptor (Image Mask 1)"="ROI Descriptor COLOR", "ROI Descriptor (Color Classification 1)"="ROI Descriptor COLOR") -> ("Image Out"=w485:T5, "error out"=w483:errorcluster, "Classes (Color Classification 1)"=w486:string[])  [unwired: 21 in]
            n49 = Index Array(array=w486, index=0) -> (element=w494:string)
            n50 = local read "Ball index"() -> (w488:i32)
            n51 = Decimal String To Number(string=w494) -> (number=w489:i32)  [unwired: 2 in, 1 out]
            "Color" <- w489
            n52 = Replace Array Subset(array=w490, new element=w489, index=w488) -> (w491:i32[])
            n53 = Bundle By Name "Bundle By Name"(cluster=w496, "qsm.Analyzed image ref"=w485, "Color class"=w489, "___Test___"=w491) -> (w495:T7)
          }
          frame "(image) show" {
            # "Show image -- Select from among the available image buffers to show on the main image display; use a selector tree or case structure."
            n54 = Unbundle By Name "Unbundle By Name"(w499) -> ("show analyzed"=w498:bool)
            n55 = Unbundle By Name "Unbundle By Name"(w501) -> ("qsm.Analyzed image ref"=w504:T5, "qsm.Webcam image ref"=w503:T5)
            n56 = Select(t=w504, s=w498, f=w503) -> (s? t:f=→"image display":T5)
          }
          frame "(ball) Shape detection" {
            # "Shape detection"
            # "Expansion State A"
            n57 = Unbundle By Name(w519) -> ("qsm.Webcam image ref"=w521:T5)
            n58 = call "Vision Assistant"("Image In"=w521, "error in"=w522, "Circle Descriptor (Shape Detection 1)"="Circle Descriptor (Shape Detection 1)") -> ("Image Out"=w520:T5, "error out"=w517:errorcluster, "Circles Calibrated (Shape Detection 1)"=w515:T2, "Number of Matches (Shape Detection 1)"=→"Number of Matches (Shape Detection 1)":i32)  [unwired: 21 in]
            "Circles Calibrated (Shape Detection 1)" <- w515
            n59 = Index Array(array=w515, index=0) -> (element=w511:T23)
            n60 = Unbundle By Name(w511) -> ("Position"=w510:cluster{"X":sgl, "Y":sgl}, "Radius"=→"CircleRadius":dbl)
            n61 = Unbundle(w510) -> ("X"=w509:sgl, "Y"=w508:sgl)
            n62 = To Double Precision Float(number=w509) -> (double precision float=→"curX":dbl)
            n63 = To Double Precision Float(number=w508) -> (double precision float=→"curY":dbl)
            n64 = Bundle By Name(cluster=w519, "qsm.Analyzed image ref"=w520) -> (w518:T7)
          }
          frame "(ball) Calc ball indx" {
            n65 = control-ref of="Ball index"() -> (w523:refnum<vi>)
            n66 = control-ref of="Number of Matches (Shape Detection 1)"() -> (w525:refnum<vi>)
            n67 = call "Ball Index (SubVI).vi"("Ball index"="Ball index", "reference in"=w523, "Digital in"=w525) -> ()  [unwired: 9 in]
          }
          frame "(ball) Calculate ROI" {
            n68 = local read "Number of Matches (Shape Detection 1)"() -> (w539:i32)
            n69 = Greater Than 0?(x=w539) -> (x > 0?=w536:bool)
            n70 = local read "curX"() -> (w538:dbl)
            n71 = local read "curY"() -> (w537:dbl)
            n72 = control-ref of="CircleRadius"() -> (w531:refnum<vi>)
            n73 = local read "ROI Descriptor COLOR"() -> (w529:T1)
            n74 = call "Ball ROI (SubVI).vi"("ROI Descriptor COLOR Mask"=w529, "divider (circle)"="divider (circle)", "curY"=w537, "curX"=w538, "Boolean"=w536, "Digital in"=w531) -> ("x1"=→"x1 (circle)":i32, "y0"=→"y0 (circle)":i32, "x0"=→"x0 (circle)":i32, "ROI Descriptor COLOR Mask out"=w530:T1, "y1"=→"y1 (circle)":i32)  [unwired: 1 in]
            n75 = local write "ROI Descriptor COLOR"(w530) -> ()
            "error out 2" <- w543
          }
          frame "X align" {
            # "Align"
            # "Expansion State B"
            n76 = case shown="True" "Align X - t, Y - f" {
              tunnel: w546 -> [w550 w566]
              frame False {
                # "Bck"
                # "Fwd"
                # "Y align"
                n77 = local read "curY"() -> (w558:dbl)
                n78 = local read "Range"() -> (w553:dbl)
                n79 = Subtract(x="defY", y=w558) -> (x-y=w552:dbl)
                n80 = Multiply(x=w553, y=-1.0) -> (x*y=w551:dbl)
                n81 = Greater?(x=w552, y=w553) -> (0:w554:bool)
                n82 = Less?(x=w552, y=w551) -> (x < y?=w555:bool)
                n83 = Not Or(1:w555, 2:w554) -> (0:w556:bool)
                "Y is in range" <- w556
                n84 = case shown="True" w556 {
                  tunnel: w550 -> [_ w559]
                  frame False {
                  }
                  frame True {
                    n85 = local read "X is in range"() -> (w560:bool)
                    n86 = case shown="False" w560 {
                      tunnel: w559 -> [_ w562]
                      frame False {
                        n87 = local write "Align X - t, Y - f"(TRUE ("X - t, Y - f")) -> ()
                      }
                      frame True {
                        w563 = T21 [enum."Wait", enum."(image) get", enum."(myRIO) clean up", enum."(qsm) shutdown"] items=["(qsm) schedule", "(qsm) initialize", "(qsm) release", "(qsm) clean up", "(qsm) shutdown", "(myRIO) initialize", "(myRIO) clean up", "(myRIO) update ports", "(image) get", "(image) analyze", "(image) show", "(ball) Shape detection", "(ball) Calc ball indx", "(ball) Calculate ROI", "X align", "Wait", "Grab", "(pattern) Find Square", "(pattern) Calculate ROI", "(pattern) Analyze pattern", "(joystick) Joystick control", "Wait for button"] ("task")
                        n88 = call "enqueue_states.vi"("task"=w563, "queue in"=w562) -> ()  [unwired: 7 in, 2 out]
                      }
                    }
                  }
                }
                n89 = local write "Left-"(w555) -> ()
                n90 = local write "Left+"(w554) -> ()
                n91 = local write "Right+"(w554) -> ()
                n92 = local write "Right-"(w555) -> ()
              }
              frame True {
                # "X align"
                # "Right"
                # "Left"
                n93 = local read "curX"() -> (w567:dbl)
                n94 = Subtract(x="defX", y=w567) -> (x-y=w574:dbl)
                n95 = Multiply(x="Range", y=-1.0) -> (x*y=w573:dbl)
                n96 = Greater?(x=w574, y="Range") -> (0:w564:bool)
                n97 = Less?(x=w574, y=w573) -> (x < y?=w565:bool)
                n98 = Not(x=w565) -> (.not. x?=w570:bool)
                n99 = Not(x=w565) -> (.not. x?=w571:bool)
                n100 = And(x=w571, y=w570) -> (x .and. y?=w569:bool)
                "X is in range" <- w569
                n101 = case shown="True" w569 {
                  tunnel: w566 -> [_ w576]
                  frame False {
                  }
                  frame True {
                    n102 = local read "Y is in range"() -> (w577:bool)
                    n103 = case shown="False" w577 {
                      tunnel: w576 -> [_ w579]
                      frame False {
                        n104 = local write "Align X - t, Y - f"(FALSE ("X - t, Y - f")) -> ()
                      }
                      frame True {
                        w580 = T21 [enum."Wait", enum."(image) get", enum."(myRIO) clean up", enum."(qsm) shutdown"] items=["(qsm) schedule", "(qsm) initialize", "(qsm) release", "(qsm) clean up", "(qsm) shutdown", "(myRIO) initialize", "(myRIO) clean up", "(myRIO) update ports", "(image) get", "(image) analyze", "(image) show", "(ball) Shape detection", "(ball) Calc ball indx", "(ball) Calculate ROI", "X align", "Wait", "Grab", "(pattern) Find Square", "(pattern) Calculate ROI", "(pattern) Analyze pattern", "(joystick) Joystick control", "Wait for button"] ("task")
                        n105 = call "enqueue_states.vi"("task"=w580, "queue in"=w579) -> ()  [unwired: 7 in, 2 out]
                      }
                    }
                  }
                }
                n106 = local write "Left-"(w564) -> ()
                n107 = local write "Left+"(w565) -> ()
                n108 = local write "Right+"(w564) -> ()
                n109 = local write "Right-"(w565) -> ()
              }
            }
          }
          frame "Wait" {
            w591 = FALSE
            # "Expansion State D"
            n110 = local read "X is in range"() -> (w589:bool)
            n111 = local read "Y is in range"() -> (w588:bool)
            n112 = local write "Left-"(w591) -> ()
            n113 = local write "Left+"(w591) -> ()
            n114 = local write "Right+"(w591) -> ()
            n115 = local write "Right-"(w591) -> ()
            n116 = And(x=w589, y=w588) -> (x .and. y?=w590:bool)
            n117 = case shown="True" w590 {
              tunnel: w587 -> [w594 w599]
              tunnel: [w594 w599] -> w586
              tunnel: w585 -> [w593 w600]
              tunnel: [w593 w600] -> w584
              tunnel: w583 -> [w592 w595]
              tunnel: [w592 w598] -> w582
              tunnel: w581 -> [_ w596]
              frame False {
              }
              frame True {
                w597 = T21 [enum."(image) get", enum."(image) analyze", enum."(image) show", enum."(myRIO) update ports", enum."Grab", enum."Wait"] items=["(qsm) schedule", "(qsm) initialize", "(qsm) release", "(qsm) clean up", "(qsm) shutdown", "(myRIO) initialize", "(myRIO) clean up", "(myRIO) update ports", "(image) get", "(image) analyze", "(image) show", "(ball) Shape detection", "(ball) Calc ball indx", "(ball) Calculate ROI", "X align", "Wait", "Grab", "(pattern) Find Square", "(pattern) Calculate ROI", "(pattern) Analyze pattern", "(joystick) Joystick control", "Wait for button"] ("task")
                n118 = call "enqueue_states.vi"("task"=w597, "error in"=w595, "queue in"=w596) -> ("error out"=w598:errorcluster)  [unwired: 6 in, 1 out]
              }
            }
          }
          frame "Grab" {
            # "Expansion State E"
            n119 = flat-sequence {
              tunnel: w602 -> [w607]
              tunnel: [w606] -> w601
              frame #0 {
                n120 = xnode "M_PWM 2"("Duty Cycle"=0.5, "Frequency [Hz]"=400.0, "error in (no error)"=w607) -> ("error out"=w608:errorcluster)
                n121 = xnode "Digital output (1 sample) 3"("M+ (B/DIO5 (Pin 21))"="M+ (onGrab)", "error in (no error)"=w608) -> ("error out"=w606:errorcluster)
                n122 = Wait (ms)(milliseconds to wait="grab time (ms)") -> ()  [unwired: 1 out]
              }
            }
          }
          frame "(pattern) Find Square" {
            # "analyzed image buffer is\ncreated during the first\ncall of the Vision\nAssistant Express VI *only*\nwhen \"Create Destination\nImage\" option is enabled"
            # "Expansion State F"
            n123 = Unbundle By Name "Unbundle By Name"(w684) -> ("qsm.Webcam image ref"=w689:T5)
            n124 = call "Vision Assistant3"("Image In"=w689, "error in"=w685) -> ("Image Out"=w682:T5, "error out"=w686:errorcluster, "Calibrated Matches (Geometric Matching 1)"=→"Calibrated Matches (Geometric Matching 1)":T3[], "Number of Matches (Geometric Matching 1)"=→"Number of Matches (Geometric Matching 1)":i32)  [unwired: 22 in]
            n125 = Bundle By Name(cluster=w684, "qsm.Analyzed image ref"=w682) -> (w683:T7)
          }
          frame "(pattern) Calculate ROI" {
            # "Expansion State G"
            n126 = local read "Number of Matches (Geometric Matching 1)"() -> (w691:i32)
            n127 = Greater Than 0?(x=w691) -> (x > 0?=w696:bool)
            n128 = case shown="True" w696 {
              tunnel: [w698 w739] -> w694
              tunnel: w693 -> [w697 w738]
              frame False {
                w699 = 0 ("index")
                # "\"Black screen\", if no squares found"
                n129 = Unbundle By Name(w697) -> ("ROI Descriptor (Image Mask 1).Contours"=w706:T24)
                n130 = Index Array(array=w706, index=0) -> (element=w709:T25)
                n131 = Unbundle By Name(w709) -> ("Coordinates"=w708:i32[])
                n132 = Replace Array Subset(array=w708, new element #1=w699, index #1=0 ("index"), new element #2=w699, index #2=1 ("index"), new element #3=w699, index #3=2 ("index"), new element #4=w699, index #4=3 ("index")) -> (w710:i32[])
                n133 = Bundle By Name(cluster=w709, "Coordinates"=w710) -> (w711:T25)
                n134 = Replace Array Subset(array=w706, new element=w711, index=0) -> (w707:T24)
                n135 = Bundle By Name(cluster=w697, "ROI Descriptor (Image Mask 1).Contours"=w707) -> (w698:T7)
              }
              frame True {
                n136 = local read "Scale"() -> (w714:sgl)
                n137 = local read "Calibrated Matches (Geometric Matching 1)"() -> (w743:T3[])
                n138 = Index Array(array=w743, index=0) -> (element=w741:T3)
                n139 = Unbundle By Name(w741) -> ("Position"=w740:cluster{"x":sgl, "y":sgl}, "Scale"=→"Scale":sgl)
                n140 = Divide(x=w714, y="y") -> (x/y=w713:sgl)
                n141 = Unbundle(w740) -> ("x"=w733:sgl, "y"=w732:sgl)
                n142 = Unbundle By Name(w738) -> ("ROI Descriptor (Image Mask 1).Contours"=w736:T24)
                n143 = Index Array(array=w736, index=0) -> (element=w725:T25)
                n144 = Unbundle By Name(w725) -> ("Coordinates"=w727:i32[])
                n145 = Subtract(x=w733, y=w713) -> (x-y=w731:sgl)
                n146 = Subtract(x=w732, y=w713) -> (x-y=w730:sgl)
                n147 = Add(x=w733, y=w713) -> (x+y=w728:sgl)
                n148 = Add(x=w732, y=w713) -> (x+y=w729:sgl)
                n149 = To Long Integer(number=w731) -> (32bit integer=w722:i32)
                "x0" <- w722
                n150 = To Long Integer(number=w730) -> (32bit integer=w721:i32)
                "y0" <- w721
                n151 = To Long Integer(number=w728) -> (32bit integer=w720:i32)
                "x1" <- w720
                n152 = To Long Integer(number=w729) -> (32bit integer=w719:i32)
                "y1" <- w719
                n153 = Replace Array Subset(array=w727, new element #1=w722, index #1=0 ("index"), new element #2=w721, index #2=1 ("index"), new element #3=w720, index #3=2 ("index"), new element #4=w719, index #4=3 ("index")) -> (w724:i32[])
                n154 = Bundle By Name(cluster=w725, "Coordinates"=w724) -> (w723:T25)
                n155 = Replace Array Subset(array=w736, new element=w723, index=0) -> (w735:T24)
                n156 = Bundle By Name(cluster=w738, "ROI Descriptor (Image Mask 1).Contours"=w735) -> (w739:T7)
              }
            }
          }
          frame "(pattern) Analyze pattern" {
            n157 = Unbundle By Name(w749) -> ("qsm.Webcam image ref"=w753:T5, "ROI Descriptor (Image Mask 1)"=w747:T1)
            n158 = call "Vision Assistant4"("Image In"=w753, "error in"=w751, "ROI Descriptor (Image Mask 1)"=w747, "ROI Descriptor (Particle Classification 1)"=w747) -> ("Image Out"=w752:T5, "error out"=w750:errorcluster, "Class (Particle Classification 1)"=w745:string)  [unwired: 21 in]
            "Class (Particle Classification 1)" <- w745
            n159 = Decimal String To Number(string=w745) -> (number=w744:i32)  [unwired: 2 in, 1 out]
            n160 = Bundle By Name(cluster=w749, "qsm.Analyzed image ref"=w752, "Pattern class"=w744) -> (w748:T7)
          }
          frame "(joystick) Joystick control" {
            # "Cross (-1 - none; 0 - up; 90 - right; 180 - down; 270 - left)"
            n161 = shared-variable "My Computer\\KeyLibrary.lvlib\\Cross"() -> (w778:i32)  [unwired: 1 in, 1 out]
            n162 = shared-variable "My Computer\\KeyLibrary.lvlib\\A"() -> (w773:bool)  [unwired: 1 in, 1 out]
            n163 = shared-variable "My Computer\\KeyLibrary.lvlib\\B"() -> (w772:bool)  [unwired: 1 in, 1 out]
            n164 = shared-variable "My Computer\\KeyLibrary.lvlib\\X"() -> (w771:bool)  [unwired: 1 in, 1 out]
            n165 = shared-variable "My Computer\\KeyLibrary.lvlib\\Y"() -> (w762:bool)  [unwired: 1 in, 1 out]
            n166 = Equal?(x=w778, y=1) -> (x = y?=w766:bool)
            n167 = Equal?(x=w778, y=90) -> (x = y?=w765:bool)
            n168 = Equal?(x=w778, y=180) -> (x = y?=w764:bool)
            n169 = Equal?(x=w778, y=270) -> (x = y?=w763:bool)
            n170 = case shown="False" w762 {
              selector: w762 -> [w793 _]
              tunnel: w761 -> [w791 w829]
              tunnel: [w790 w829] -> w760
              frame False {
                n171 = Not(x=w793) -> (.not. x?=w792:bool)
                n172 = xnode "LED 3"("LED3"=w792, "error in (no error)"=w791) -> ("error out"=w790:errorcluster)
              }
              frame True {
              }
            }
            n173 = Or(x=w763, y=w771) -> (x .or. y?=w774:bool)
            n174 = local write "G-"(w774) -> ()
            n175 = Or(x=w766, y=w762) -> (x .or. y?=w777:bool)
            n176 = Or(x=w764, y=w773) -> (x .or. y?=w776:bool)
            n177 = local write "M+"(w777) -> ()
            n178 = local write "M-"(w776) -> ()
            n179 = Or(x=w765, y=w772) -> (x .or. y?=w775:bool)
            n180 = local write "G+"(w775) -> ()
            n181 = shared-variable "My Computer\\KeyLibrary.lvlib\\Forward"() -> (w757:bool)  [unwired: 1 in, 1 out]
            n182 = shared-variable "My Computer\\KeyLibrary.lvlib\\Left"() -> (w755:bool)  [unwired: 1 in, 1 out]
            n183 = shared-variable "My Computer\\KeyLibrary.lvlib\\Back"() -> (w756:bool)  [unwired: 1 in, 1 out]
            n184 = shared-variable "My Computer\\KeyLibrary.lvlib\\Right"() -> (w754:bool)  [unwired: 1 in, 1 out]
            n185 = Build Array(w757, w755, w756, w754) -> (w758:bool[])
            n186 = Or Array Elements(Boolean array=w758) -> (logical OR=w759:bool)
            n187 = case shown="True" w759 {
              selector: w759 -> [w781 _]
              tunnel: w757 -> [_ w789]
              tunnel: w756 -> [_ w788]
              tunnel: w755 -> [_ w783]
              tunnel: w754 -> [_ w782]
              frame False {
                n188 = local write "Right+"(w781) -> ()
                n189 = local write "Right-"(w781) -> ()
                n190 = local write "Left+"(w781) -> ()
                n191 = local write "Left-"(w781) -> ()
              }
              frame True {
                n192 = Or(x=w789, y=w782) -> (x .or. y?=w787:bool)
                n193 = Or(x=w788, y=w782) -> (x .or. y?=w784:bool)
                n194 = Or(x=w788, y=w783) -> (x .or. y?=w786:bool)
                n195 = Or(x=w783, y=w789) -> (x .or. y?=w785:bool)
                n196 = local write "Left+"(w787) -> ()
                n197 = local write "Left-"(w786) -> ()
                n198 = local write "Right+"(w785) -> ()
                n199 = local write "Right-"(w784) -> ()
              }
            }
          }
          frame "Wait for button" {
            n200 = while {
              stop <- w836 stop-if-true
              n201 = local read "Stop"() -> (w835:bool)
              n202 = Or(x="Look at ball", y=w835) -> (x .or. y?=w836:bool)
            }
            n203 = local write "Look at ball"(FALSE ("Look at ball")) -> ()
          }
        }
        n204 = Merge Errors(w49, w48) -> (w26:errorcluster)
        n205 = xnode "LED"("LED0"="x = y?", "error in (no error)"=w26) -> ("error out"=w25:errorcluster)
        n206 = Merge Errors(w17, w25) -> (w53:errorcluster)
        n207 = Unbundle By Name(w21) -> ("Pattern class"=w24:i32, "___Test___"=w16:i32[])
        "___Test___" <- w16
        n208 = local read "Number of Matches (Shape Detection 1)"() -> (w23:i32)
        n209 = local read "Ball index"() -> (w14:i32)
        n210 = Index Array(array=w16, index=w14) -> (element=w15:i32)
        n211 = Equal?(x=w24, y=w15) -> (x = y?=w18:bool)
        n212 = local write "x = y?"(w18) -> ()
        n213 = Greater Than 0?(x=w23) -> (x > 0?=w22:bool)
        n214 = case shown="True" w22 {
          tunnel: [w64 w70] -> w20
          tunnel: w21 -> [w63 w70]
          frame False {
            n215 = Unbundle By Name(w63) -> ("___Test___"=w60:i32[])
            n216 = for {
              N: 5 -> [w68]
              tunnel: [w69] -> w62
              tunnel: w60 -> [w66]
              n217 = Decrement(x=w68) -> (x-1=w67:i32)
              n218 = Replace Array Subset(array=w66, new element=20, index=w67) -> (w69:i32[])
            }
            n219 = Bundle By Name(cluster=w63, "___Test___"=w62) -> (w64:T7)
          }
          frame True {
          }
        }
      }
    }
    frame #1 {
      w840 = FALSE ("X is in range")
      n220 = call <vilib>:"Simple Error Handler.vi"("error in (no error)"=w839) -> ("error out"=w838:errorcluster)  [unwired: 4 in, 4 out]
      "error out" <- w838
      n221 = local write "X is in range"(w840) -> ()
      n222 = local write "Y is in range"(w840) -> ()
      n223 = local write "Stop"(w840) -> ()
      n224 = local write "Look at ball"(w840) -> ()
      n225 = local write "x = y?"(w840) -> ()
      n226 = local write "Ball index"(1 ("Ball index")) -> ()
    }
  }
  n227 = call <vilib>:"Reset myRIO.vi"("error in (no error)"=w7) -> ()  [unwired: 10 in, 1 out]
